vi "Custom Device CORE.vi"(8 "error in (no error)":errorcluster, 11 "CD Wizard - Internal Data":T1={"Common Information"={"CD Name"="InlineAsync", "CD Target Folder"=path "C:/Users/rsparks/Desktop/Test1", "CD Execution Mode"=enum."Inline HW Interface", "CD GUID"="", "Max Occurrences"=1}, "Extra Pages"=[{"Page Name"="Page 0", "Page GUID"="0-000000000000000-00000000000-000"}, {"Page Name"="Page11", "Page GUID"=""}, {"Page Name"="Page 2", "Page GUID"="22222222-222222222-2222222"}, {"Page Name"="Page33", "Page GUID"=""}, {"Page Name"="Page4", "Page GUID"="44444444-44444444444-4444444"}], "References"={"System Explorer Library"=refnum, "Shared Library"=refnum, "Engine Library"=refnum}, "Menu Settings"={"Insert CD in submenu"=FALSE, "Parent Menu Name"=""}}) -> (0 "error out":errorcluster)   [LabVIEW 2015]
doc: "This VI is the Core VI for the Custom Device Wizard.\n\nWritten by:\nStephan Daunke\n\nDate:\n2014/01/27\n\nCompany:\nNational Instruments Germany GmbH"
uses:
  TypDef/CD Wizard - Internal data.ctl
  TypDef/CD Wizard - Execution Mode.ctl
  TypDef/CD Wizard - Extra Page Name and GUID.ctl
  TypDef/CD Wizard - Action.ctl
  Constants/Constants TypDef/Common.ctl
  Constants/Constants TypDef/Utility folder.ctl
  Constants/Constants TypDef/CD Shared lvlib.ctl
  TypDef/Add Item - Type.ctl
  Constants/Constants TypDef/CD System Explorer lvlib.ctl
  Constants/Constants TypDef/CD Engine lvlib.ctl
  Constants/Constants TypDef/Build Spec System Explorer.ctl
  Constants/Constants TypDef/Build Spec Engine.ctl
  Constants/Common.vi
  Constants/Utility folder.vi
  Constants/CD Shared lvlib.vi
  Constants/CD System Explorer lvlib.vi
  Constants/CD Engine lvlib.vi
  <vilib>/Utility/config.llb/Write Key (String).vi
  <vilib>/Utility/config.llb/Write Key (Path).vi
  Constants/Build Spec System Explorer.vi
  Constants/Build Spec Engine.vi
  <vilib>/Utility/config.llb/NI_LVConfig.lvlib
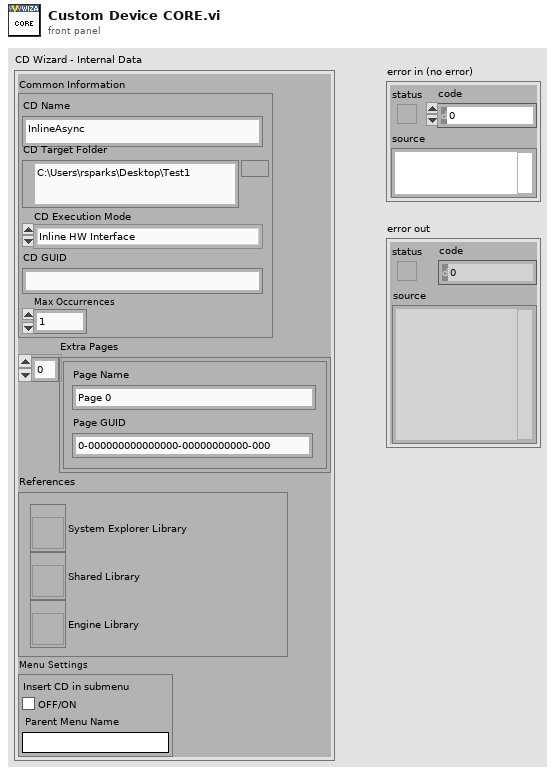
[diagram p1: front panel]
types:
  T1 = typedef "CD Wizard - Internal data.ctl" = cluster{"Common Information":cluster{"CD Name":string, "CD Target Folder":path, "CD Execution Mode":T2, "CD GUID":string, "Max Occurrences":u32}, "Extra Pages":T3[], "References":cluster{"System Explorer Library":refnum<vi>, "Shared Library":refnum<vi>, "Engine Library":refnum<vi>}, "Menu Settings":cluster{"Insert CD in submenu":bool, "Parent Menu Name":string}}
  T2 = typedef "CD Wizard - Execution Mode.ctl" = enum16{"Asynchronous", "Inline HW Interface", "Inline Model Interface", "Inline Timing and Sync", "Asynchronous Timing and Sync"}
  T3 = typedef "CD Wizard - Extra Page Name and GUID.ctl" = cluster{"Page Name":string, "Page GUID":string}
  T4 = typedef "CD Wizard - Action.ctl" = enum16{"Initialize", "Project - Create Custom Device folder", "Project - Copy Readme.rtf into the CD folder", "PC - Create GUID for each extra page", "PC-Utility - Create folder and copy -Copy .LLB to NI VeriStand dir-", "PC-Utility - Change -Copy .LLB to NI VeriStand dir-", "PC-Shared - Create folder and copy Constants.vi", "PC-Shared - Change Constants.vi content", "PC-Shared - Create library", "PC-Shared - Add folders and VIs to library", "PC-System Explorer - Create folder and copy templates", "PC-System Explorer - Create extra pages", "PC-System Explorer - Create library", "PC-System Explorer - Add folders and VIs to library", "PC-Engine - Create folder and copy the RT Template", "PC-Engine - Create library", "PC-Engine - Add virtual folders and VIs to library", "PC-XML - Create and change file", "PC-Help - Copy HTML Files", "Project - Read project file content", "Project - Edit Utility section", "Project - Edit XML section", "Project - Edit Engine Library section", "Project - Edit Shared Library section", "Project - Edit System Explorer Library section", "Project - Edit Custom Device Name", "Project - Edit System Explorer LLB Name", "Project - Edit Engine LLB OS dependent file name", "Project - Write new project file", "Shutdown"}
  T5 = typedef "Common.ctl" = enum16{"ProjectName", "TemplatesFolderName", "ProjectTemplatePathAndName", "ReadmeTemplatePathAndName", "TimingAndSyncFolderName", "CustomDeviceFolderName", "PathToTemplates"}
  T6 = typedef "Utility folder.ctl" = enum16{"Utility.FolderName", "Utility.Copy .llb to NI VeriStand dir.FileName", "Utility.Copy .llb to NI VeriStand dir.FilePathAndName", "Utility.LLB Pre Build.FilePathAndName"}
  T7 = typedef "CD Shared lvlib.ctl" = enum16{"LibraryFileName", "LibraryFolderName", "ConstantsVI.VIPathAndName", "Shared.FolderName", "Shared.Types.FolderName", "Shared.Constants.VIName", "Shared.Constants.VITemplateName", "Shared.Constants.VITemplatePathAndName", "Shared.CompiledSettings.RelativePath", "Shared.Constants.RelativePath", "Shared.CompiledSettings.Name", "Shared.CompiledSettings.Name.NoExtension", "Shared.CompiledSettings.ClusterName"}
  T8 = typedef "CD System Explorer lvlib.ctl" = enum16{"LibraryFileName", "LibraryFolderName", "System Explorer.FolderName", "System Explorer.Dynamically Called.FolderName", "System Explorer.Dynamically Called.Extra Pages.FolderName", "System Explorer.Dynamically Called.Extra Pages.TemplatePathAndName", "System Explorer.Dynamically Called.Main Page.VIName", "System Explorer.Dynamically Called.Main Page.TemplatePathAndName", "System Explorer.Dynamically Called.Initialization VI.VIName", "System Explorer.Dynamically Called.Initialization VI.TemplatePathAndName", "System Explorer.SubVI.FolderName", "System Explorer.Types.FolderName", "System Explorer.ActionVIOnCompile.VIName", "System Explorer.ExportConfigRTM.VIName"}
  T9 = typedef "CD Engine lvlib.ctl" = enum16{"LibraryFileName", "LibraryFolderName", "Engine.FolderName", "Engine.Init.FolderName", "Engine.Run.FolderName", "Engine.Shutdown.FolderName", "Types.FolderName", "Engine.RT Driver VI.TemplatePath", "Engine.RT Driver VI.FileName", "Engine.RTStateVariables.Name", "Engine.RTStateVariables.Name.NoExtension", "Engine.Async.NameExtension", "Engine.Async.TemplateName"}
  T10 = typedef "Build Spec System Explorer.ctl" = enum16{"Destinations.LLBFileName"}
  T11 = typedef "Build Spec Engine.ctl" = enum16{"Destinations.LLBWindowsFileName", "Destinations.LLBVxWorksFileName", "Destinations.LLBPharlapFileName", "Destinations.LLBLinuxARMFileName", "Destinations.LLBLinux64FileName"}
  T12 = enum16{"open", "replace", "create", "open or create", "replace or create", "replace or create with confirmation"}
  T13 = typedef "Add Item - Type.ctl" = string
  T14 = typedef "NI_LVConfig.lvlib/Config Data RefNum.ctl" = refnum<k1>
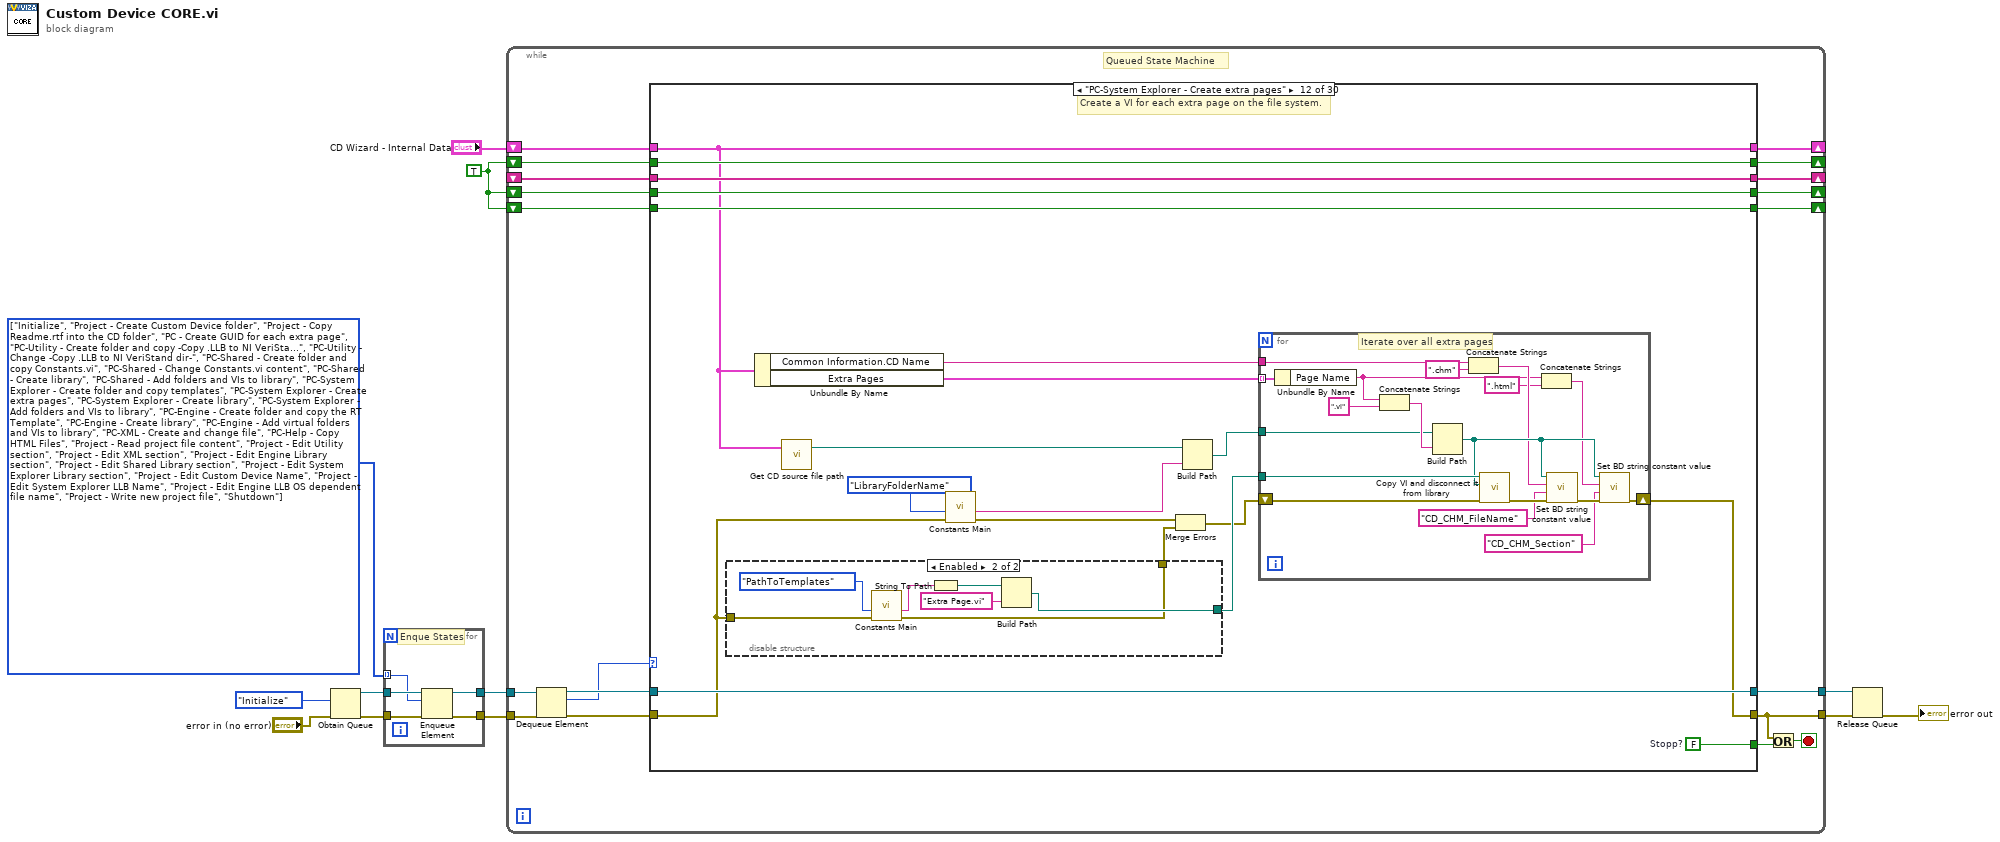
[diagram p0: block diagram]
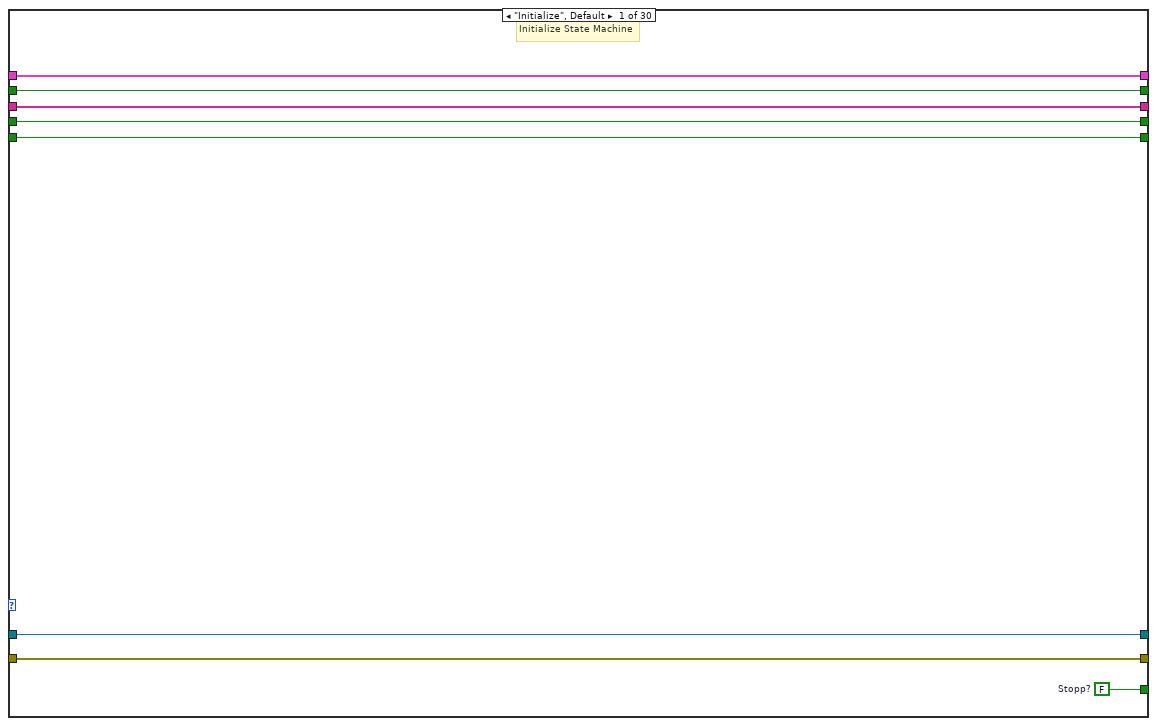
[diagram p2: hidden frame]
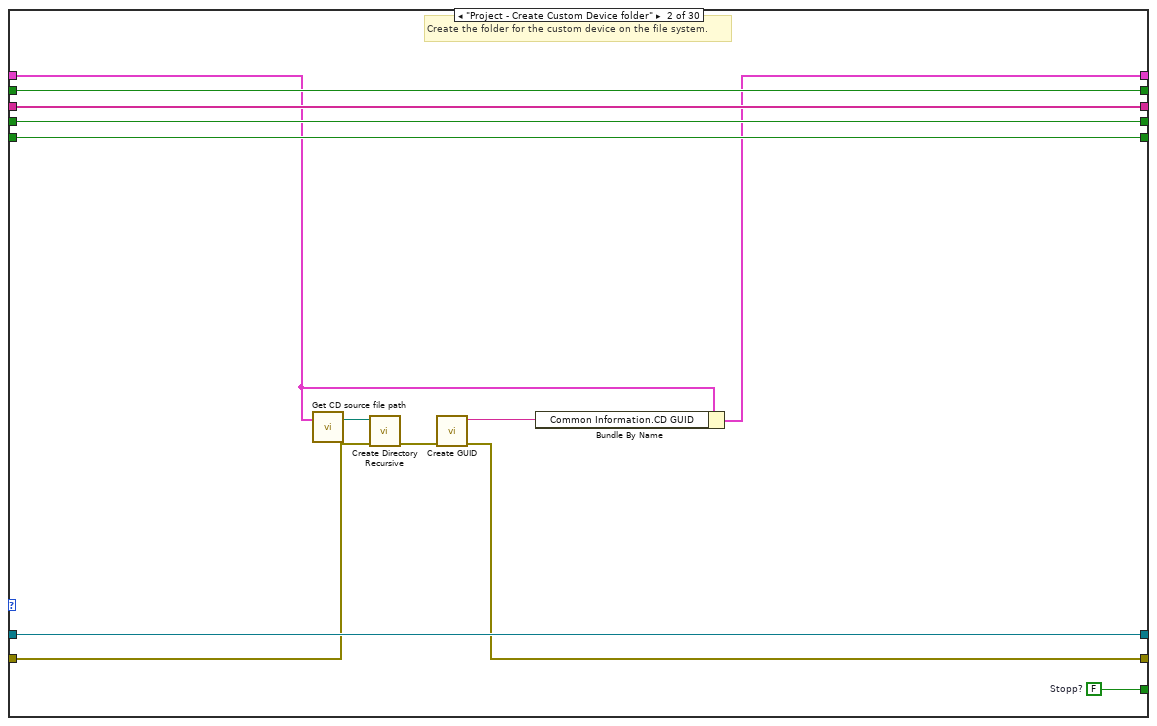
[diagram p3: hidden frame]
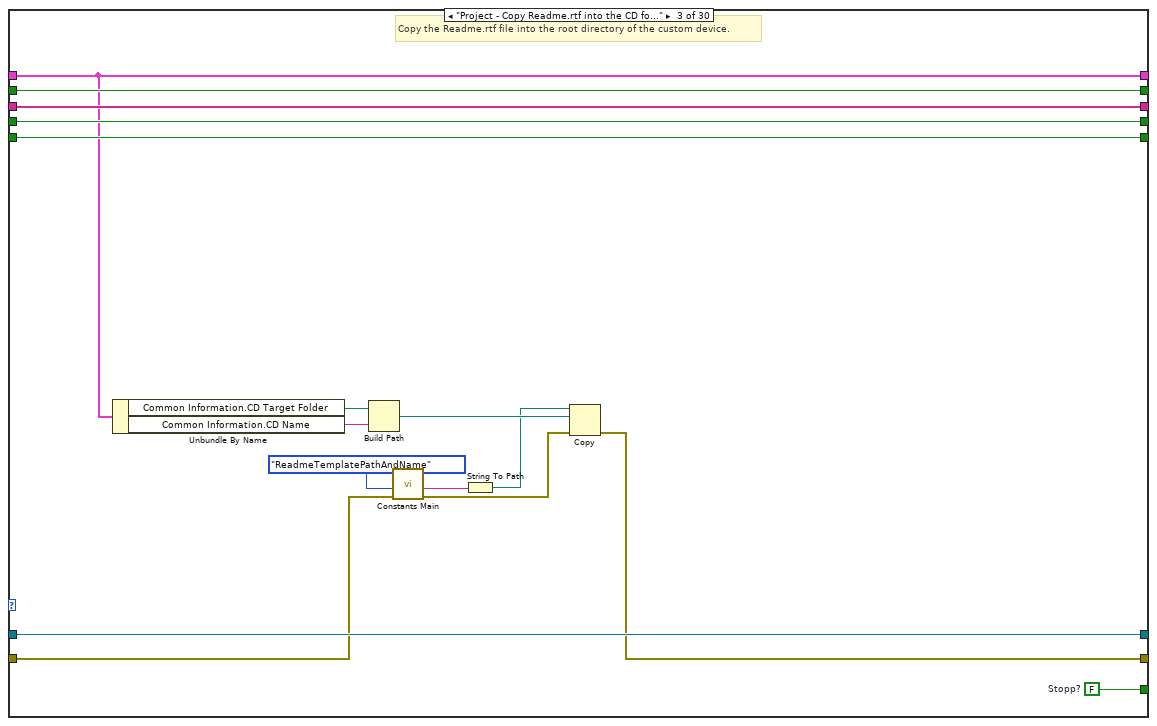
[diagram p4: hidden frame]
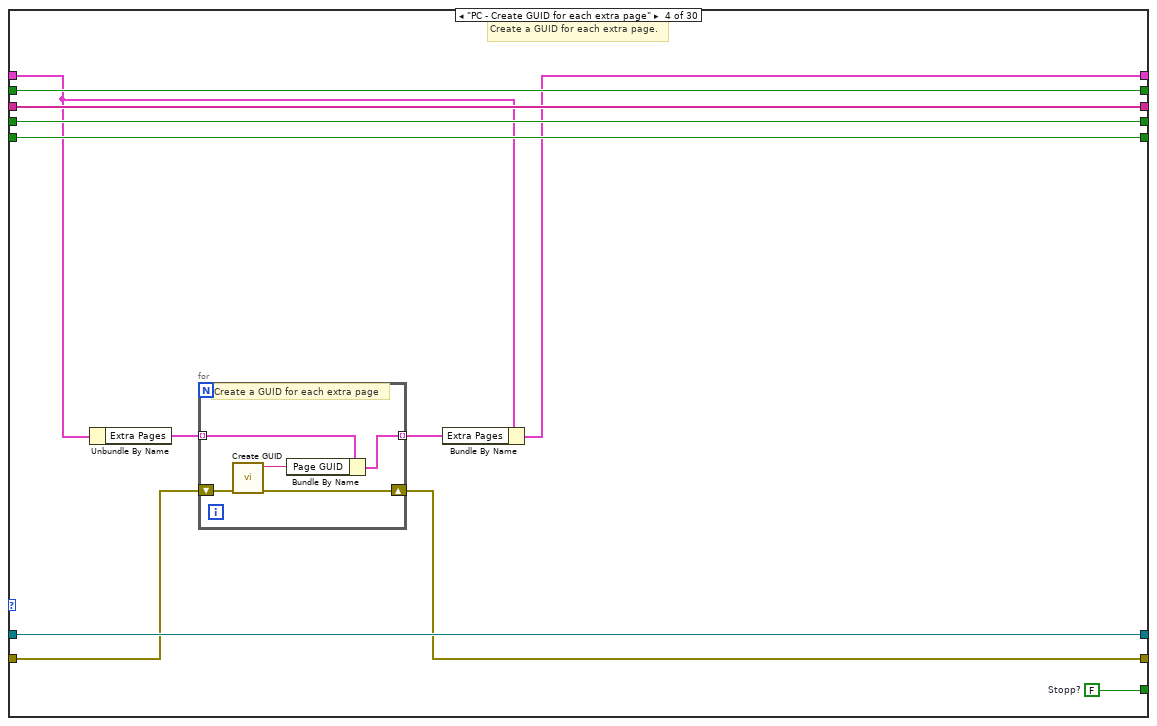
[diagram p5: hidden frame]
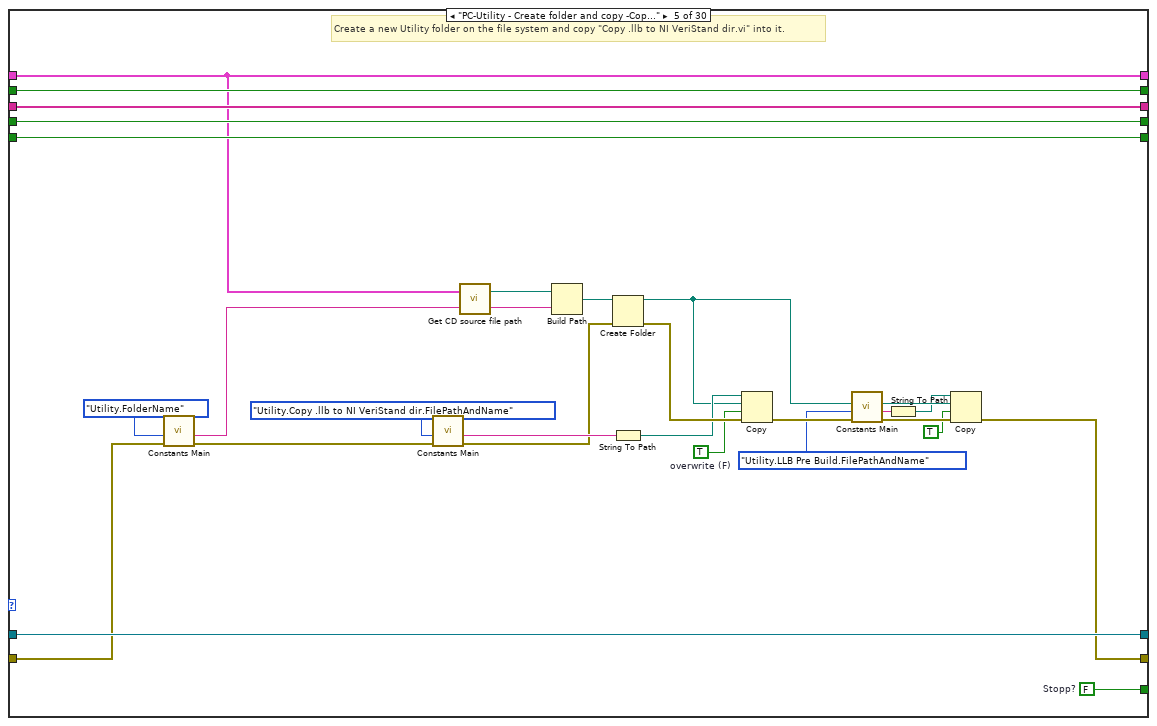
[diagram p6: hidden frame]
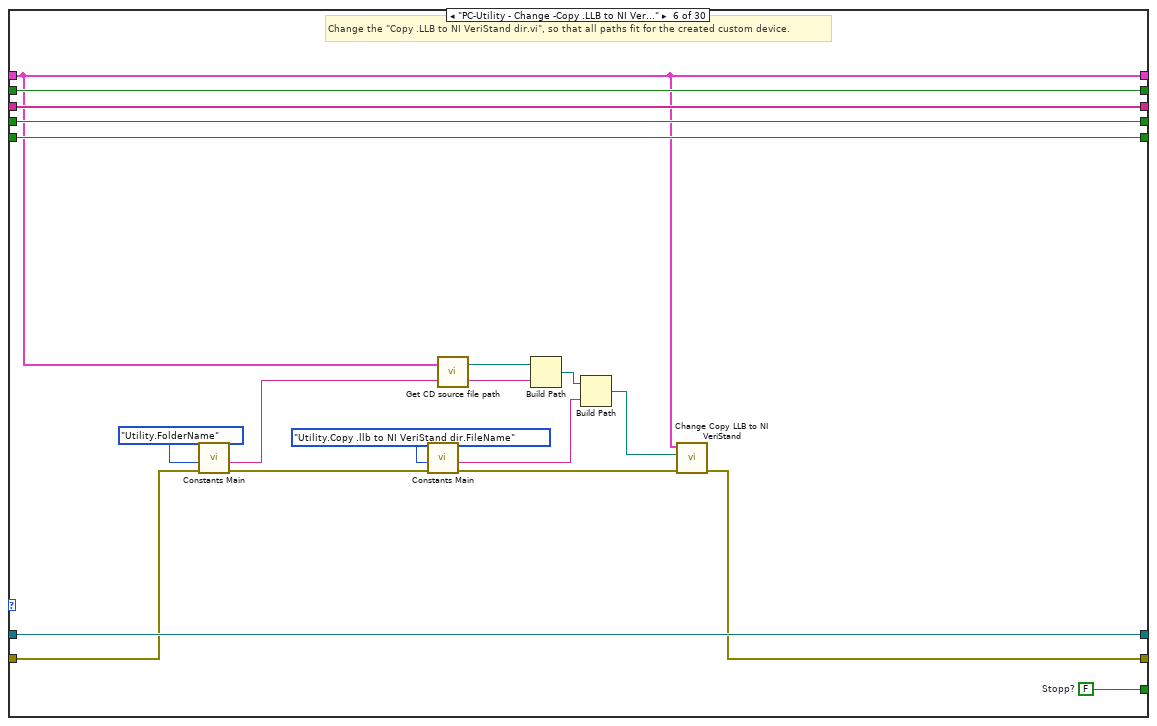
[diagram p7: hidden frame]
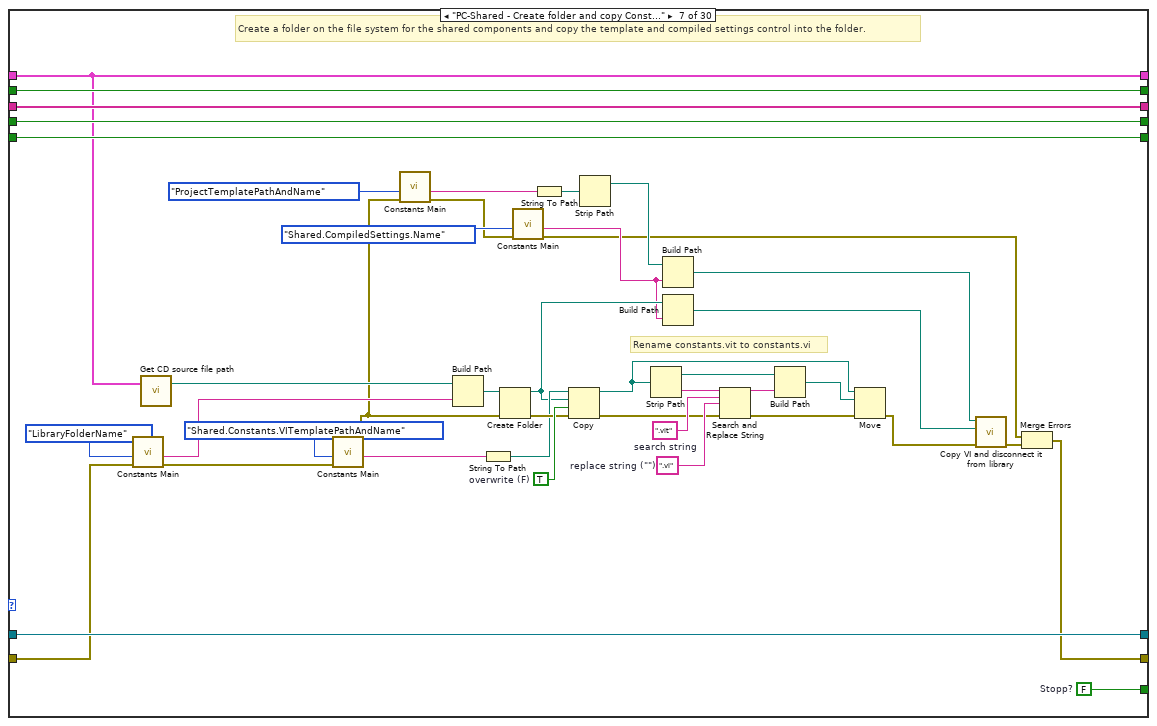
[diagram p8: hidden frame]
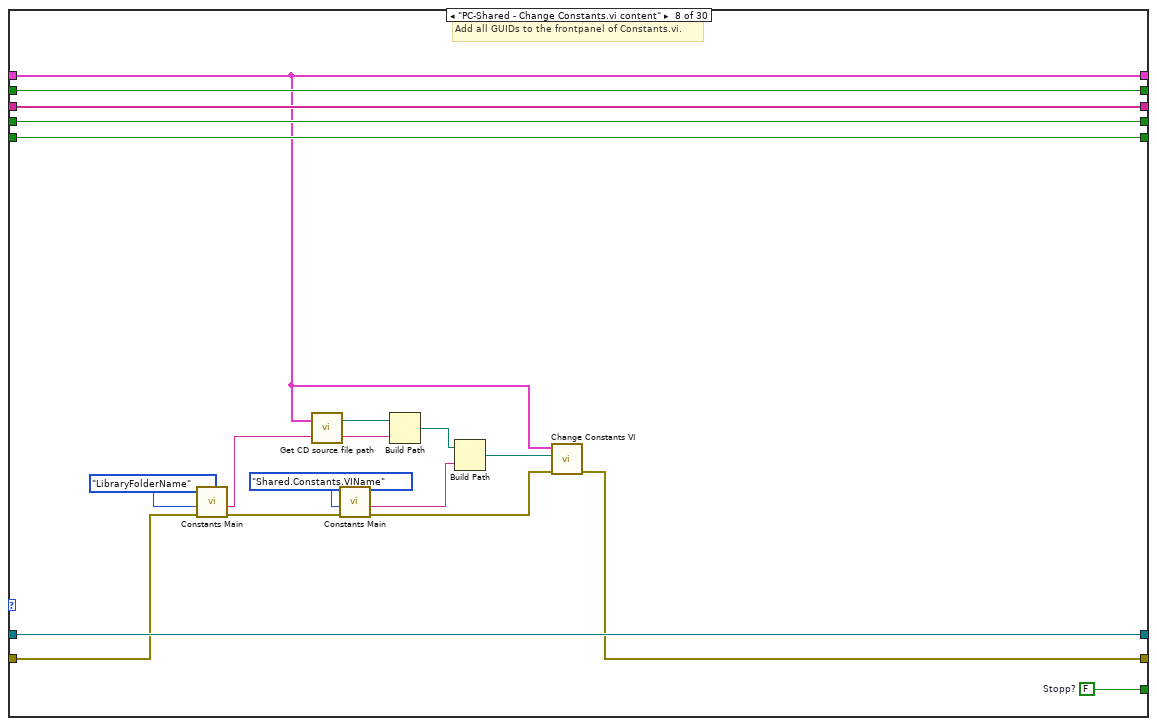
[diagram p9: hidden frame]
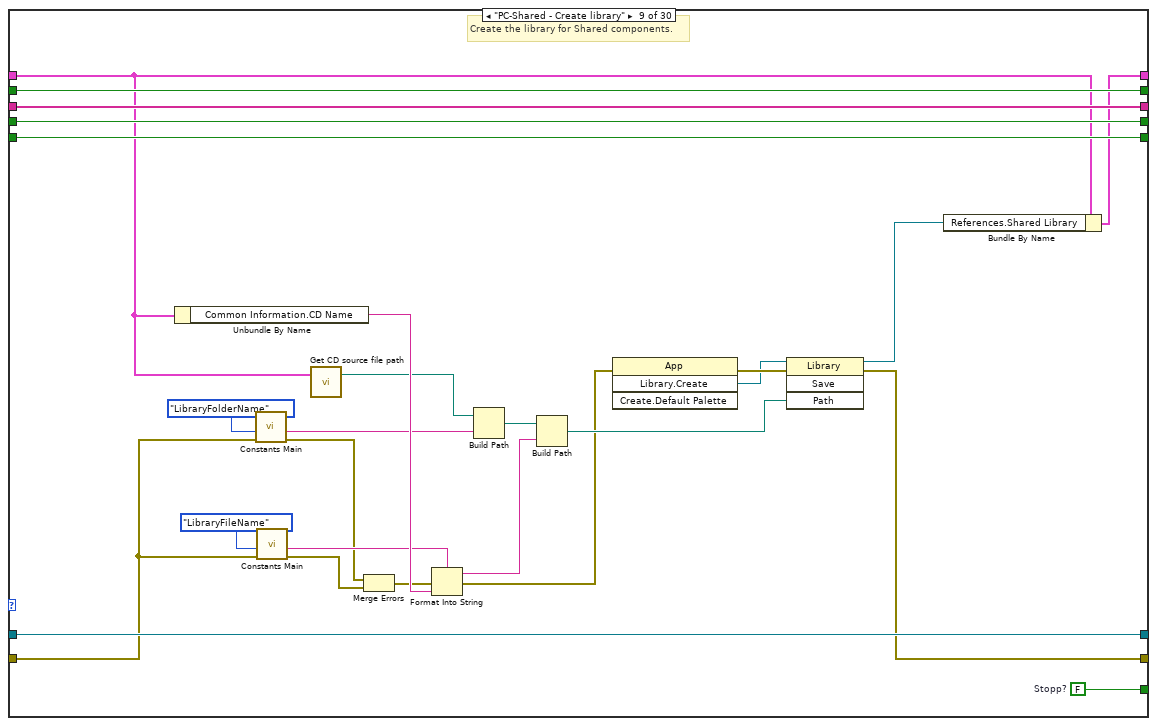
[diagram p10: hidden frame]
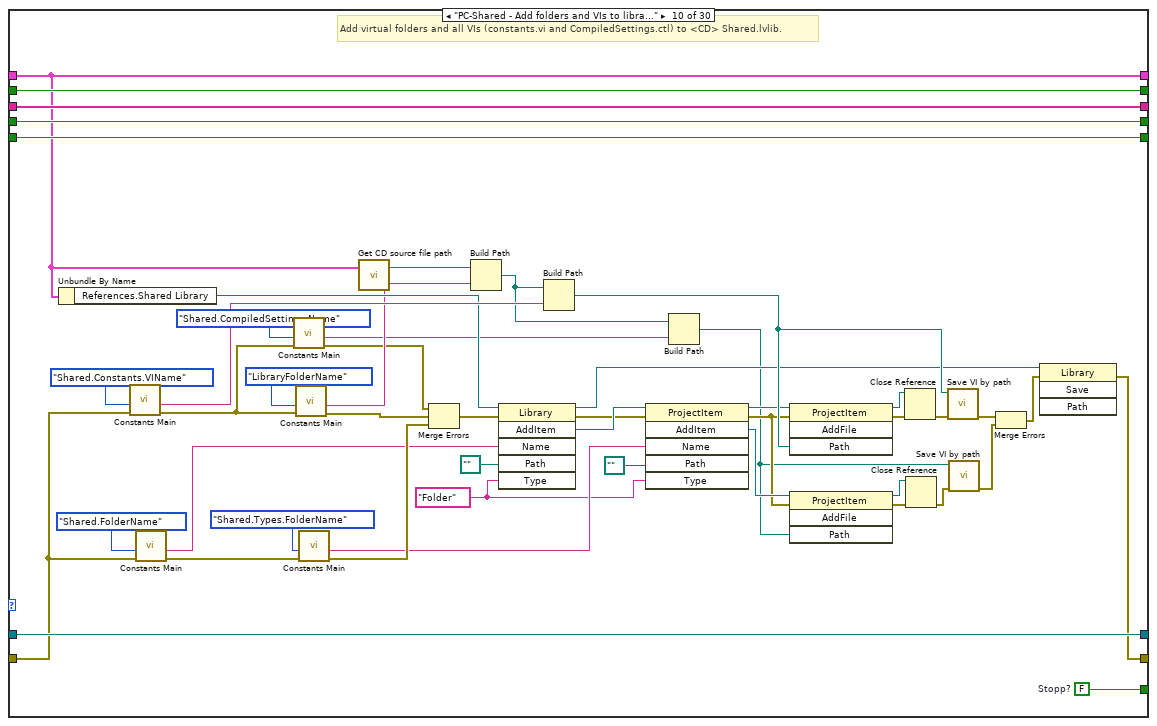
[diagram p11: hidden frame]
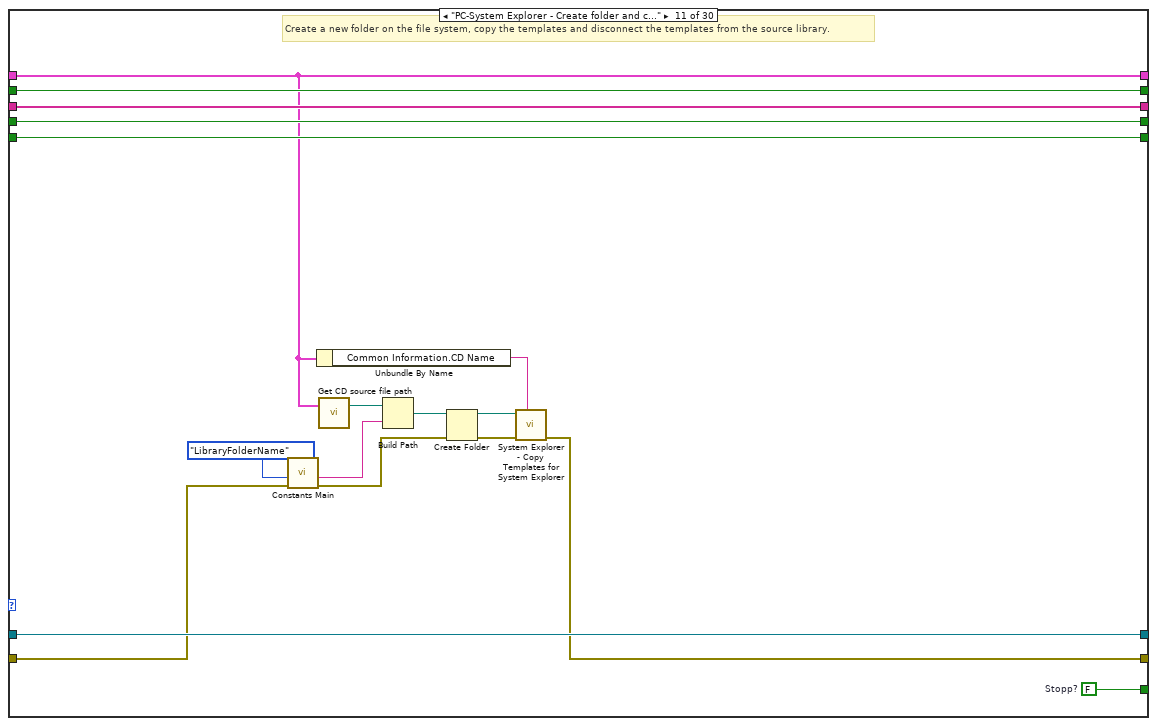
[diagram p12: hidden frame]
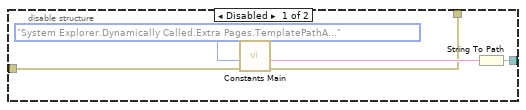
[diagram p13: hidden frame]
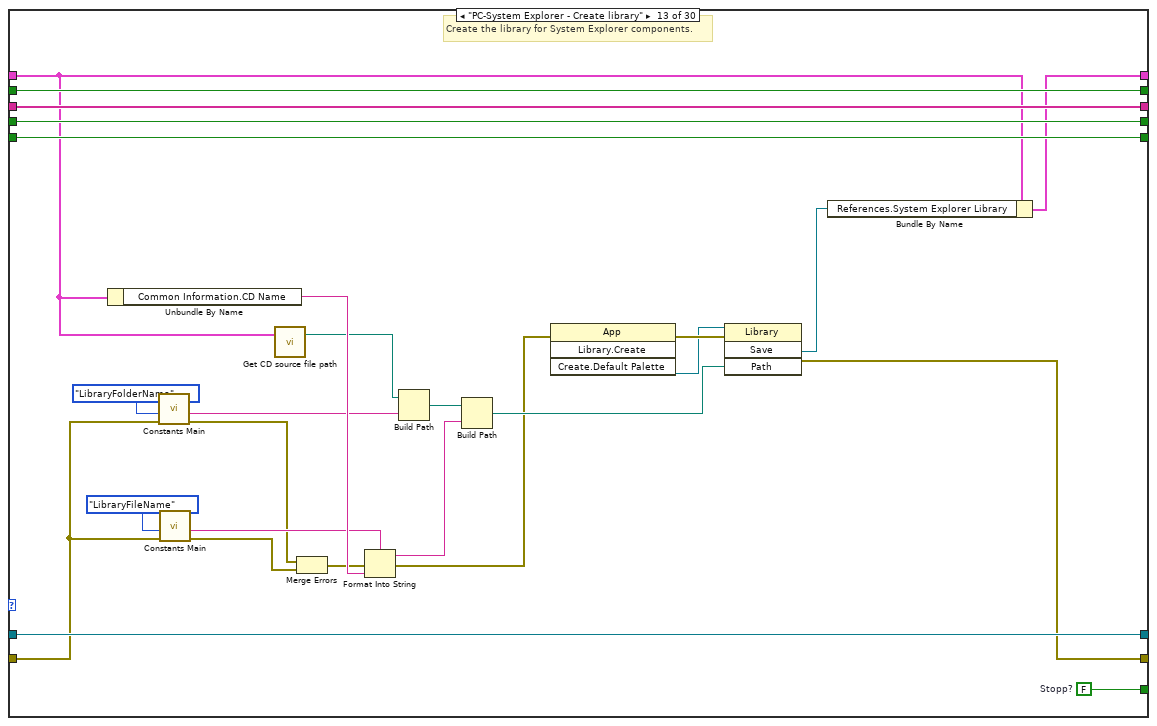
[diagram p14: hidden frame]
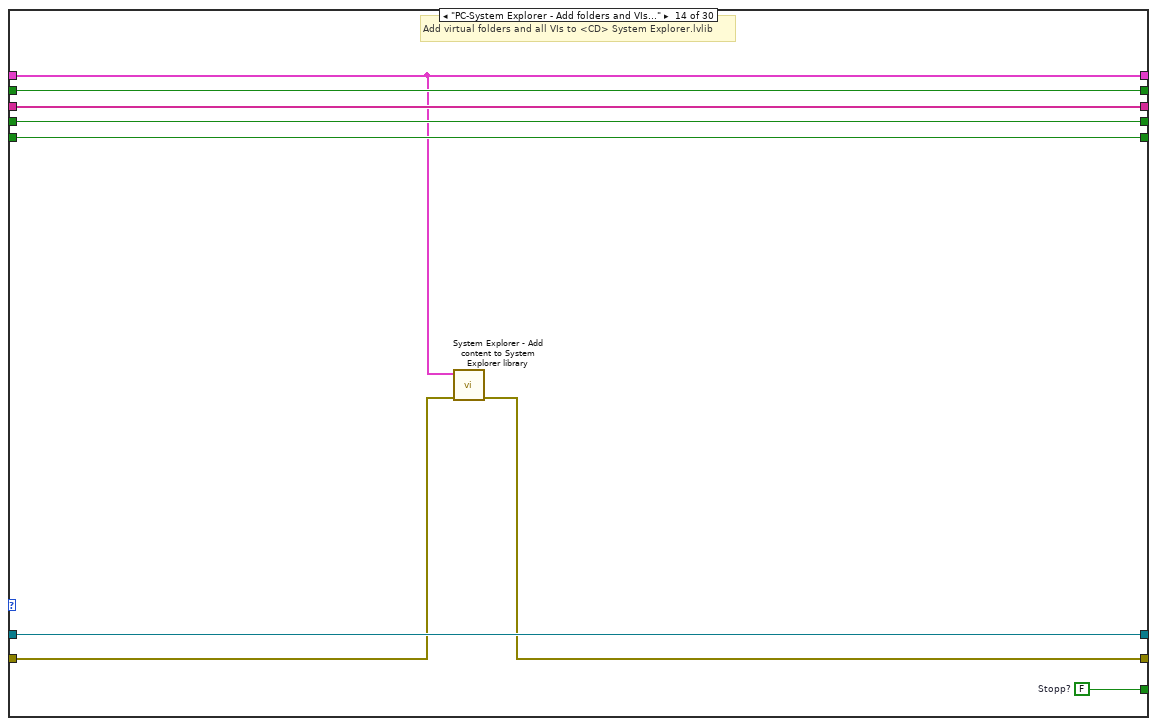
[diagram p15: hidden frame]
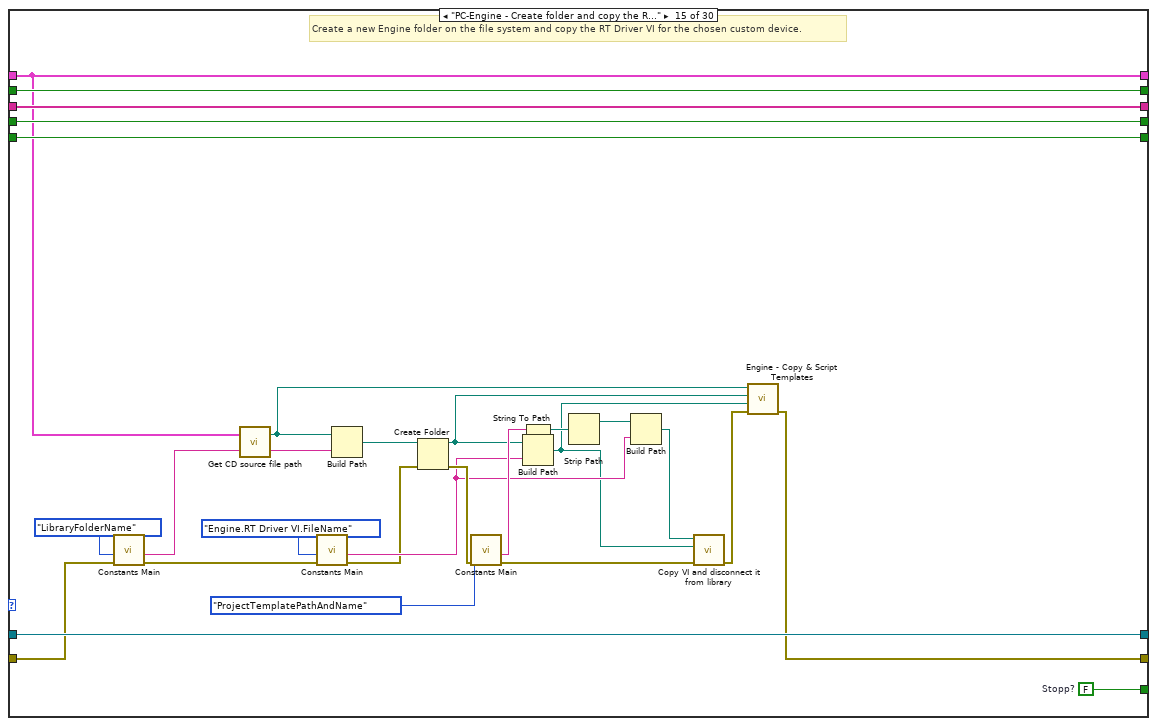
[diagram p16: hidden frame]
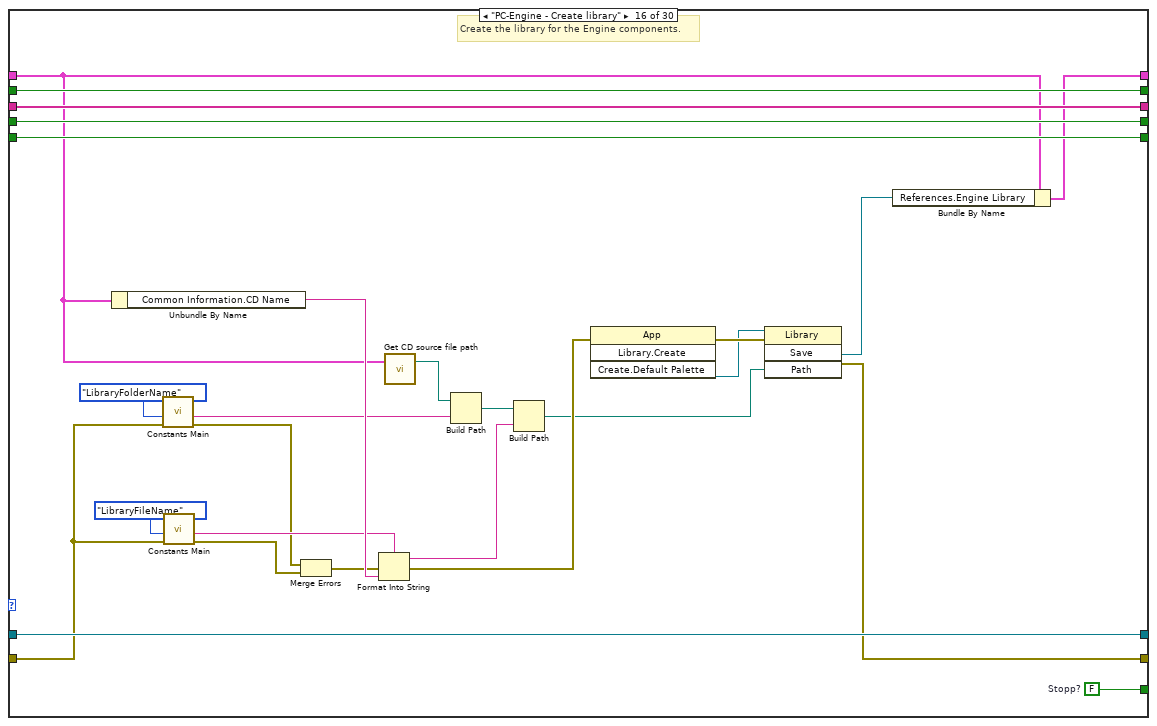
[diagram p17: hidden frame]
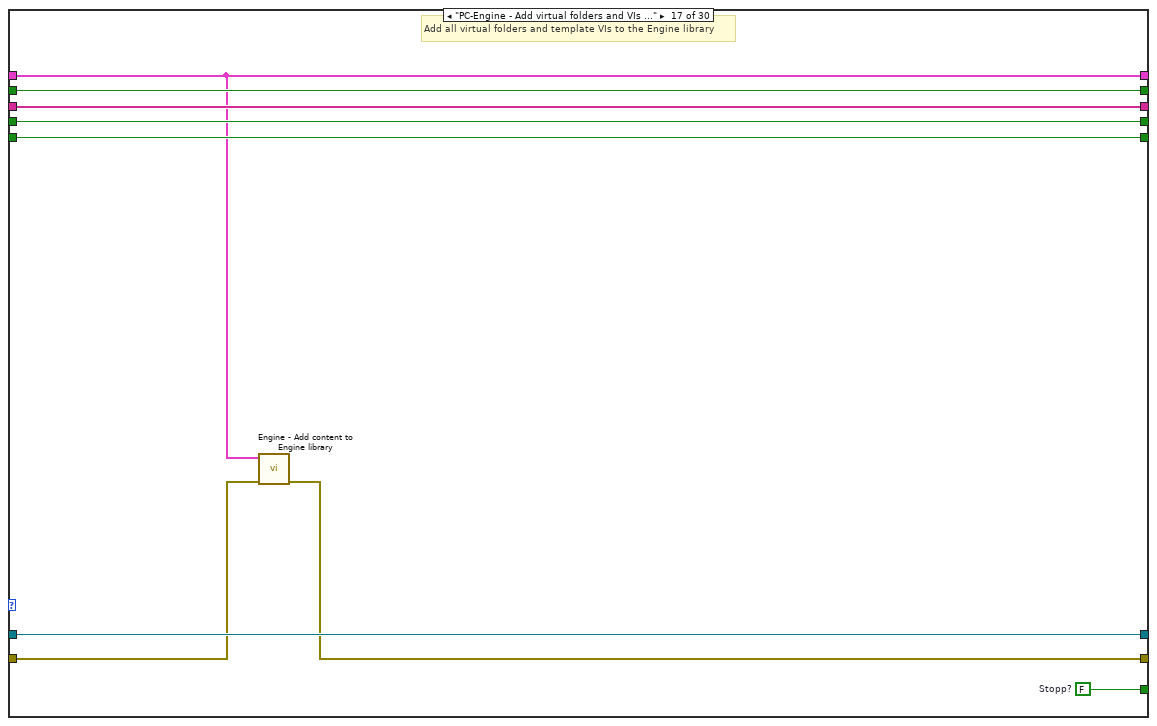
[diagram p18: hidden frame]
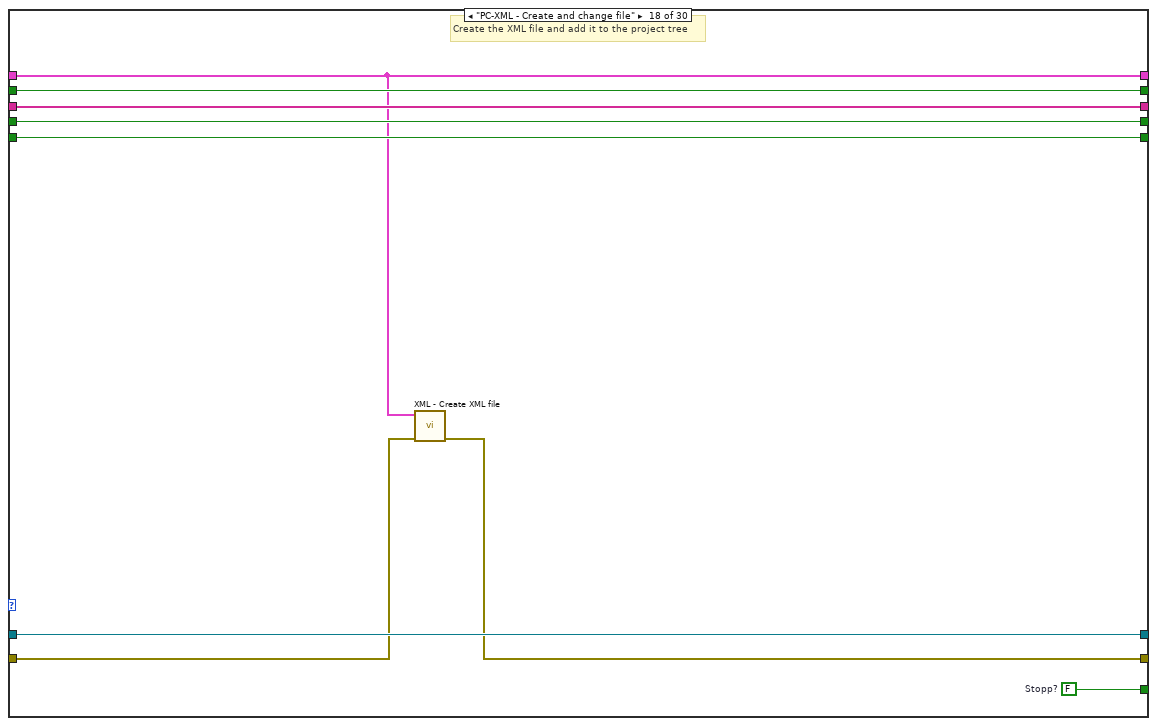
[diagram p19: hidden frame]
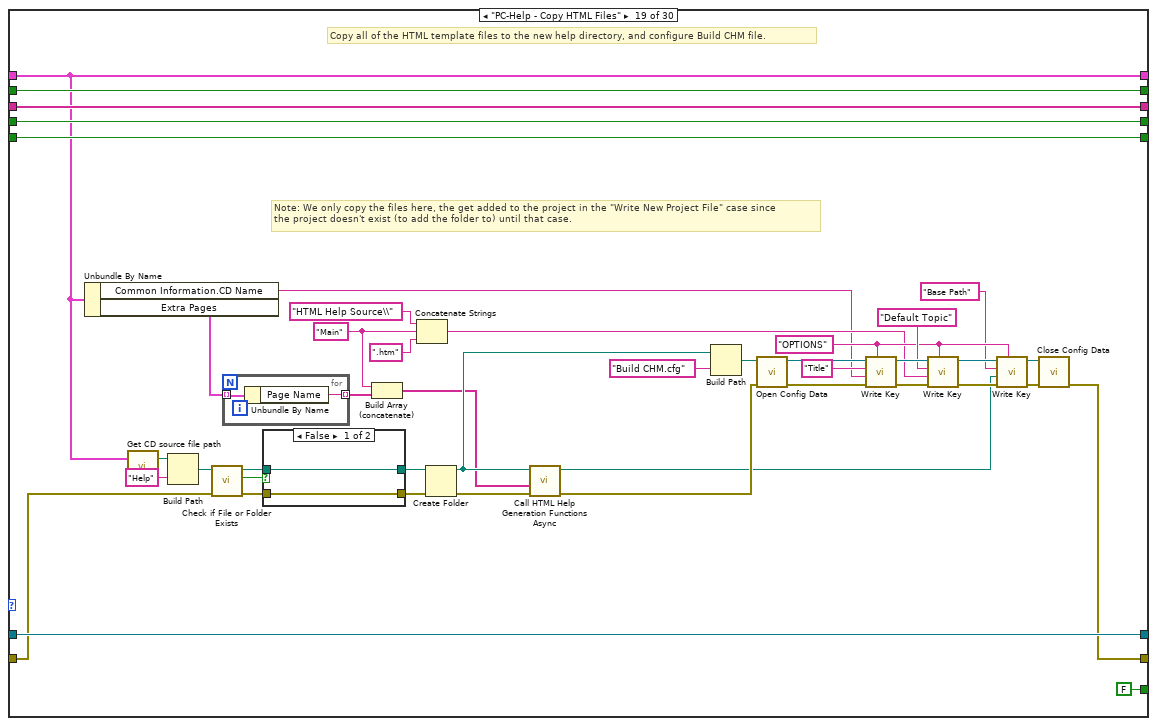
[diagram p20: hidden frame]
diagram:
  w3 = TRUE
  w6 = T4[] [enum."Initialize", enum."Project - Create Custom Device folder", enum."Project - Copy Readme.rtf into the CD folder", enum."PC - Create GUID for each extra page", enum."PC-Utility - Create folder and copy -Copy .LLB to NI VeriStand dir-", enum."PC-Utility - Change -Copy .LLB to NI VeriStand dir-", enum."PC-Shared - Create folder and copy Constants.vi", enum."PC-Shared - Change Constants.vi content", enum."PC-Shared - Create library", enum."PC-Shared - Add folders and VIs to library", enum."PC-System Explorer - Create folder and copy templates", enum."PC-System Explorer - Create extra pages", enum."PC-System Explorer - Create library", enum."PC-System Explorer - Add folders and VIs to library", enum."PC-Engine - Create folder and copy the RT Template", enum."PC-Engine - Create library", enum."PC-Engine - Add virtual folders and VIs to library", enum."PC-XML - Create and change file", enum."PC-Help - Copy HTML Files", enum."Project - Read project file content", enum."Project - Edit Utility section", enum."Project - Edit XML section", enum."Project - Edit Engine Library section", enum."Project - Edit Shared Library section", enum."Project - Edit System Explorer Library section", enum."Project - Edit Custom Device Name", enum."Project - Edit System Explorer LLB Name", enum."Project - Edit Engine LLB OS dependent file name", enum."Project - Write new project file", enum."Shutdown"] items=["Initialize", "Project - Create Custom Device folder", "Project - Copy Readme.rtf into the CD folder", "PC - Create GUID for each extra page", "PC-Utility - Create folder and copy -Copy .LLB to NI VeriStand dir-", "PC-Utility - Change -Copy .LLB to NI VeriStand dir-", "PC-Shared - Create folder and copy Constants.vi", "PC-Shared - Change Constants.vi content", "PC-Shared - Create library", "PC-Shared - Add folders and VIs to library", "PC-System Explorer - Create folder and copy templates", "PC-System Explorer - Create extra pages", "PC-System Explorer - Create library", "PC-System Explorer - Add folders and VIs to library", "PC-Engine - Create folder and copy the RT Template", "PC-Engine - Create library", "PC-Engine - Add virtual folders and VIs to library", "PC-XML - Create and change file", "PC-Help - Copy HTML Files", "Project - Read project file content", "Project - Edit Utility section", "Project - Edit XML section", "Project - Edit Engine Library section", "Project - Edit Shared Library section", "Project - Edit System Explorer Library section", "Project - Edit Custom Device Name", "Project - Edit System Explorer LLB Name", "Project - Edit Engine LLB OS dependent file name", "Project - Write new project file", "Shutdown"]
  n1 = Obtain Queue(element data type=CD_Wizard_-_Action."Initialize", error in (no error)="error in (no error)") -> (queue out=w10:refnum<queue>, error out=w9:errorcluster)  [unwired: 3 in, 1 out]
  n2 = for {
    tunnel: w10 -> [w17]
    tunnel: w9 -> [w16]
    tunnel: [w15] -> w8
    tunnel: [w14] -> w7
    tunnel: w6 -> [w13] mode=indexing
    # "Enque States"
    n3 = Enqueue Element(queue=w17, element=w13, error in (no error)=w16) -> (queue out=w15:refnum<queue>, error out=w14:errorcluster)  [unwired: 1 in, 1 out]
  }
  n4 = while {
    tunnel: w8 -> [w36]
    tunnel: w7 -> [w35]
    tunnel: [w21] -> w4
    tunnel: [w32] -> w11
    shift-right: [w27] -> _
    shift-left: "CD Wizard - Internal Data" -> [w31]
    shift-right: [w26] -> _
    shift-left: w3 -> [w30]
    shift-right: [w25] -> _
    shift-left: _ -> [w29]
    shift-right: [w24] -> _
    shift-left: w3 -> [w28]
    shift-right: [w23] -> _
    shift-left: w3 -> [w20]
    stop <- w22 stop-if-true
    # "Queued State Machine"
    n5 = Dequeue Element(queue=w36, error in (no error)=w35) -> (queue out=w34:refnum<queue>, element=w19:T4, error out=w33:errorcluster)  [unwired: 1 in, 1 out]
    n6 = case shown="\"PC-System Explorer - Create extra pages\"" w19 {
      tunnel: w34 -> [w44 w57 w73 w85 w117 w135 w177 w195 w221 w269 w286 w305 w361 w370 w397 w423 w432 w441 w484 w511 w533 w563 w581 w604 w643 w670 w694 w740 w791 w799]
      tunnel: w33 -> [w39 w47 w62 w79 w102 w123 w171 w181 w198 w241 w278 w289 w345 w365 w383 w405 w427 w436 w457 w497 w516 w555 w576 w587 w622 w666 w686 w712 w782 w798]
      tunnel: [w44 w57 w73 w85 w117 w135 w177 w195 w221 w269 w286 w305 w361 w370 w397 w423 w432 w441 w484 w511 w533 w563 w581 w604 w643 w670 w694 w740 w791 w799] -> w32
      tunnel: [w39 w50 w64 w78 w91 w122 w137 w190 w197 w240 w274 w299 w337 w364 w374 w401 w426 w435 w456 w502 w526 w559 w575 w599 w626 w665 w690 w721 w772 w798] -> w21
      tunnel: w31 -> [w38 w49 w66 w76 w100 w120 w165 w179 w201 w242 w271 w298 w343 w363 w387 w407 w425 w434 w452 w508 w529 w556 w574 w583 w623 w661 w684 w733 w783 w797]
      tunnel: w30 -> [w43 w56 w72 w84 w116 w134 w176 w194 w220 w268 w285 w304 w360 w369 w396 w422 w431 w440 w483 w495 w532 w562 w580 w603 w642 w669 w693 w739 w788 w796]
      tunnel: w29 -> [w42 w55 w71 w83 w115 w133 w175 w193 w219 w267 w284 w303 w359 w368 w395 w421 w430 w439 w482 _ w528 w558 w573 w588 w624 w663 w681 w722 w775 w795]
      tunnel: w28 -> [w40 w54 w70 w82 w114 w132 w174 w192 w218 w266 w283 w302 w358 w367 w394 w420 w429 w438 w481 w510 w531 w561 w579 w602 w641 w668 w692 w738 w790 w794]
      tunnel: w20 -> [w41 w53 w69 w81 w113 w131 w173 w191 w217 w265 w282 w301 w357 w366 w393 w419 w428 w437 w480 w509 w530 w560 w578 w601 w640 w667 w691 w737 w789 w793]
      tunnel: [w38 w52 w66 w75 w100 w120 w165 w179 w200 w242 w271 w298 w346 w363 w387 w406 w425 w434 w452 w508 w529 w556 w574 w583 w623 w661 w684 w733 w783 w797] -> w27
      tunnel: [w43 w56 w72 w84 w116 w134 w176 w194 w220 w268 w285 w304 w360 w369 w396 w422 w431 w440 w483 w495 w532 w562 w580 w603 w642 w669 w693 w739 w788 w796] -> w26
      tunnel: [w42 w55 w71 w83 w115 w133 w175 w193 w219 w267 w284 w303 w359 w368 w395 w421 w430 w439 w482 w501 w527 w557 w577 w600 w625 w664 w680 w703 w775 w795] -> w25
      tunnel: [w40 w54 w70 w82 w114 w132 w174 w192 w218 w266 w283 w302 w358 w367 w394 w420 w429 w438 w481 w510 w531 w561 w579 w602 w641 w668 w692 w738 w790 w794] -> w24
      tunnel: [w41 w53 w69 w81 w113 w131 w173 w191 w217 w265 w282 w301 w357 w366 w393 w419 w428 w437 w480 w509 w530 w560 w578 w601 w640 w667 w691 w737 w789 w793] -> w23
      tunnel: [w37 w45 w58 w74 w99 w118 w163 w178 w196 w235 w272 w288 w336 w362 w382 w398 w424 w433 FALSE ("Stopp?") w494 w518 w550 w572 w582 w621 w660 w679 w720 w770 w792] -> w18
      frame "Initialize", Default {
        w37 = FALSE  # Stopp?
        # "Initialize State Machine"
      }
      frame "Project - Create Custom Device folder" {
        w45 = FALSE  # Stopp?
        # "Create the folder for the custom device on the file system."
        n7 = call "Get CD source file path.vi"("CD Wizard - Internal Data"=w49) -> ("CD Source file path"=w48:path)  [unwired: 2 in]
        n8 = call <vilib>:"Create Directory Recursive.vi"("error in (no error)"=w47, "directory"=w48) -> ("error out"=w46:errorcluster)  [unwired: 3 in, 2 out]
        n9 = call "Create GUID.vi"("error in (no error)"=w46) -> ("error out"=w50:errorcluster, "Generated GUID"=w51:string)  [unwired: 9 in]
        n10 = Bundle By Name(cluster=w49, "Common Information.CD GUID"=w51) -> (w52:T1)
      }
      frame "Project - Copy Readme.rtf into the CD folder" {
        w58 = FALSE  # Stopp?
        # "Copy the Readme.rtf file into the root directory of the custom device."
        n11 = Unbundle By Name(w66) -> ("Common Information.CD Target Folder"=w68:path, "Common Information.CD Name"=w67:string)
        n12 = Build Path(base path=w68, name or relative path=w67) -> (appended path=w65:path)
        n13 = call-poly "Constants Main.vi"("error in (no error)"=w62, "Action"=Common."ReadmeTemplatePathAndName") -> ("error out"=w61:errorcluster, "Output"=w60:string)  [unwired: 8 in]
        n14 = String To Path(string=w60) -> (path=w59:path)
        n15 = Copy(8:w61, 10:w65, 11:w59) -> (0:w64:errorcluster)  [unwired: 1 in, 3 out]
      }
      frame "PC - Create GUID for each extra page" {
        w74 = FALSE  # Stopp?
        # "Create a GUID for each extra page."
        n16 = Unbundle By Name(w76) -> ("Extra Pages"=w80:T3[])
        n17 = for {
          tunnel: w80 -> [w90] mode=indexing
          shift-right: [w87] -> w78
          shift-left: w79 -> [w88]
          tunnel: [w86] -> w77 mode=indexing
          # "Create a GUID for each extra page"
          n18 = call "Create GUID.vi"("error in (no error)"=w88) -> ("error out"=w87:errorcluster, "Generated GUID"=w89:string)  [unwired: 9 in]
          n19 = Bundle By Name(cluster=w90, "Page GUID"=w89) -> (w86:T3)
        }
        n20 = Bundle By Name(cluster=w76, "Extra Pages"=w77) -> (w75:T1)
      }
      frame "PC-Utility - Create folder and copy -Copy .LLB to NI VeriStand dir-" {
        w99 = FALSE  # Stopp?
        w110 = TRUE  # overwrite (F)
        # "Create a new Utility folder on the file system and copy \"Copy .llb to NI VeriStand dir.vi\" into it."
        n21 = call-poly "Constants Main.vi"("error in (no error)"=w102, "Action"=Utility_folder."Utility.FolderName") -> ("error out"=w103:errorcluster, "Output"=w104:string)  [unwired: 8 in]
        n22 = call-poly "Constants Main.vi"("error in (no error)"=w103, "Action"=Utility_folder."Utility.Copy .llb to NI VeriStand dir.FilePathAndName") -> ("error out"=w106:errorcluster, "Output"=w108:string)  [unwired: 8 in]
        n23 = call "Get CD source file path.vi"("CD Wizard - Internal Data"=w100) -> ("CD Source file path"=w101:path)  [unwired: 2 in]
        n24 = Build Path(base path=w101, name or relative path=w104) -> (appended path=w112:path)
        n25 = Create Folder(path (use dialog)=w112, error in=w106) -> (created path=w98:path, error out=w111:errorcluster)  [unwired: 1 in, 1 out]
        n26 = String To Path(string=w108) -> (path=w107:path)
        n27 = Copy(8:w111, 9:w110, 10:w98, 11:w107) -> (0:w97:errorcluster)  [unwired: 3 out]
        n28 = call-poly "Constants Main.vi"("error in (no error)"=w97, "Action"=Utility_folder."Utility.LLB Pre Build.FilePathAndName") -> ("error out"=w93:errorcluster, "Output"=w95:string)  [unwired: 8 in]
        n29 = String To Path(string=w95) -> (path=w94:path)
        n30 = Copy(8:w93, 9:TRUE ("overwrite (F)"), 10:w98, 11:w94) -> (0:w91:errorcluster)  [unwired: 3 out]
      }
      frame "PC-Utility - Change -Copy .LLB to NI VeriStand dir-" {
        w118 = FALSE  # Stopp?
        # "Change the \"Copy .LLB to NI VeriStand dir.vi\", so that all paths fit for the created custom device."
        n31 = call-poly "Constants Main.vi"("error in (no error)"=w123, "Action"=Utility_folder."Utility.FolderName") -> ("error out"=w127:errorcluster, "Output"=w128:string)  [unwired: 8 in]
        n32 = call-poly "Constants Main.vi"("error in (no error)"=w127, "Action"=Utility_folder."Utility.Copy .llb to NI VeriStand dir.FileName") -> ("error out"=w124:errorcluster, "Output"=w125:string)  [unwired: 8 in]
        n33 = call "Get CD source file path.vi"("CD Wizard - Internal Data"=w120) -> ("CD Source file path"=w119:path)  [unwired: 2 in]
        n34 = Build Path(base path=w119, name or relative path=w128) -> (appended path=w126:path)
        n35 = Build Path(base path=w126, name or relative path=w125) -> (appended path=w121:path)
        n36 = call "Change Copy LLB to NI VeriStand.vi"("error in (no error)"=w124, "Copy .LLB to ... path"=w121, "CD Wizard - Internal Data"=w120) -> ("error out"=w122:errorcluster)  [unwired: 8 in]
      }
      frame "PC-Shared - Create folder and copy Constants.vi" {
        w157 = ".vi"  # replace string ("")
        w158 = ".vit"  # search string
        w163 = FALSE  # Stopp?
        w162 = TRUE  # overwrite (F)
        # "Rename constants.vit to constants.vi"
        # "Create a folder on the file system for the shared components and copy the template and compiled settings control into the folder."
        n37 = call-poly "Constants Main.vi"("error in (no error)"=w171, "Action"=CD_Shared_lvlib."LibraryFolderName") -> ("error out"=w167:errorcluster, "Output"=w169:string)  [unwired: 8 in]
        n38 = call "Get CD source file path.vi"("CD Wizard - Internal Data"=w165) -> ("CD Source file path"=w164:path)  [unwired: 2 in]
        n39 = call-poly "Constants Main.vi"("error in (no error)"=w167, "Action"=CD_Shared_lvlib."Shared.Constants.VITemplatePathAndName") -> ("error out"=w140:errorcluster, "Output"=w166:string)  [unwired: 8 in]
        n40 = call-poly "Constants Main.vi"("error in (no error)"=w140, "Action"=Common."ProjectTemplatePathAndName") -> ("error out"=w138:errorcluster, "Output"=w149:string)  [unwired: 8 in]
        n41 = Build Path(base path=w164, name or relative path=w169) -> (appended path=w172:path)
        n42 = String To Path(string=w166) -> (path=w155:path)
        n43 = Create Folder(path (use dialog)=w172, error in=w140) -> (created path=w146:path, error out=w156:errorcluster)  [unwired: 1 in, 1 out]
        n44 = call-poly "Constants Main.vi"("error in (no error)"=w138, "Action"=CD_Shared_lvlib."Shared.CompiledSettings.Name") -> ("error out"=w136:errorcluster, "Output"=w139:string)  [unwired: 8 in]
        n45 = String To Path(string=w149) -> (path=w148:path)
        n46 = Copy(8:w156, 9:w162, 10:w146, 11:w155) -> (0:w154:errorcluster, 3:w151:path)  [unwired: 2 out]
        n47 = Strip Path(path=w148) -> (stripped path=w147:path)  [unwired: 1 out]
        n48 = Strip Path(path=w151) -> (stripped path=w161:path, name=w160:string)
        n49 = Build Path(base path=w147, name or relative path=w139) -> (appended path=w145:path)
        n50 = Build Path(base path=w146, name or relative path=w139) -> (appended path=w144:path)
        n51 = Search and Replace String(input string=w160, search string=w158, replace string=w157, error in=w154) -> (result string=w159:string, error out=w153:errorcluster)  [unwired: 4 in, 2 out]
        n52 = Build Path(base path=w161, name or relative path=w159) -> (appended path=w152:path)
        n53 = Move(source path=w151, error in=w153, 10:w152) -> (error out=w143:errorcluster)  [unwired: 2 in, 2 out]
        n54 = call "Copy VI and disconnect it from library.vi"("error in (no error)"=w143, "VI Target Path"=w144, "VI Source Path"=w145) -> ("error out"=w142:errorcluster)  [unwired: 8 in]
        n55 = Merge Errors(w136, w142) -> (w137:errorcluster)
      }
      frame "PC-Shared - Change Constants.vi content" {
        w178 = FALSE  # Stopp?
        # "Add all GUIDs to the frontpanel of Constants.vi."
        n56 = call-poly "Constants Main.vi"("error in (no error)"=w181, "Action"=CD_Shared_lvlib."LibraryFolderName") -> ("error out"=w184:errorcluster, "Output"=w183:string)  [unwired: 8 in]
        n57 = call "Get CD source file path.vi"("CD Wizard - Internal Data"=w179) -> ("CD Source file path"=w180:path)  [unwired: 2 in]
        n58 = call-poly "Constants Main.vi"("error in (no error)"=w184, "Action"=CD_Shared_lvlib."Shared.Constants.VIName") -> ("error out"=w182:errorcluster, "Output"=w186:string)  [unwired: 8 in]
        n59 = Build Path(base path=w180, name or relative path=w183) -> (appended path=w189:path)
        n60 = Build Path(base path=w189, name or relative path=w186) -> (appended path=w188:path)
        n61 = call "Change Constants VI.vi"("error in (no error)"=w182, "Constants.vi path"=w188, "CD Wizard - Internal Data"=w179) -> ("error out"=w190:errorcluster)  [unwired: 8 in]
      }
      frame "PC-Shared - Create library" {
        w196 = FALSE  # Stopp?
        # "Create the library for Shared components."
        n62 = Unbundle By Name(w201) -> ("Common Information.CD Name"=w216:string)
        n63 = call-poly "Constants Main.vi"("error in (no error)"=w198, "Action"=CD_Shared_lvlib."LibraryFolderName") -> ("error out"=w209:errorcluster, "Output"=w210:string)  [unwired: 8 in]
        n64 = call-poly "Constants Main.vi"("error in (no error)"=w198, "Action"=CD_Shared_lvlib."LibraryFileName") -> ("error out"=w207:errorcluster, "Output"=w211:string)  [unwired: 8 in]
        n65 = call "Get CD source file path.vi"("CD Wizard - Internal Data"=w201) -> ("CD Source file path"=w206:path)  [unwired: 2 in]
        n66 = Merge Errors(w209, w207) -> (w208:errorcluster)
        n67 = Format Into String(format string=w211, error in=w208, w216) -> (resulting string=w214:string, error out=w202:errorcluster)  [unwired: 1 in]
        n68 = Build Path(base path=w206, name or relative path=w210) -> (appended path=w215:path)
        n69 = Build Path(base path=w215, name or relative path=w214) -> (appended path=w203:path)
        n70 = invoke class="App" method="Library.Create"(error in=w202) -> (error out=w205:errorcluster, "Create Library"=w204:refnum<vi>)  [unwired: 3 in, 2 out]
        n71 = invoke class="Library" method="Save"(reference=w204, error in=w205, "Path"=w203) -> (reference out=w199:refnum<vi>, error out=w197:errorcluster)  [unwired: 1 in, 2 out]
        n72 = Bundle By Name(cluster=w201, "References.Shared Library"=w199) -> (w200:T1)
      }
      frame "PC-Shared - Add folders and VIs to library" {
        w235 = FALSE  # Stopp?
        w248 = T13 "Folder" ("Add Item - Type")
        # "Add virtual folders and all VIs (constants.vi and CompiledSettings.ctl) to <CD> Shared.lvlib."
        n73 = Unbundle By Name(w242) -> ("References.Shared Library"=w244:refnum<vi>)
        n74 = call-poly "Constants Main.vi"("error in (no error)"=w241, "Action"=CD_Shared_lvlib."Shared.Constants.VIName") -> ("error out"=w227:errorcluster, "Output"=w263:string)  [unwired: 8 in]
        n75 = call-poly "Constants Main.vi"("error in (no error)"=w241, "Action"=CD_Shared_lvlib."Shared.FolderName") -> ("error out"=w259:errorcluster, "Output"=w237:string)  [unwired: 8 in]
        n76 = call-poly "Constants Main.vi"("error in (no error)"=w227, "Action"=CD_Shared_lvlib."Shared.CompiledSettings.Name") -> ("error out"=w226:errorcluster, "Output"=w225:string)  [unwired: 8 in]
        n77 = call-poly "Constants Main.vi"("error in (no error)"=w227, "Action"=CD_Shared_lvlib."LibraryFolderName") -> ("error out"=w238:errorcluster, "Output"=w236:string)  [unwired: 8 in]
        n78 = call-poly "Constants Main.vi"("error in (no error)"=w259, "Action"=CD_Shared_lvlib."Shared.Types.FolderName") -> ("error out"=w261:errorcluster, "Output"=w258:string)  [unwired: 8 in]
        n79 = call "Get CD source file path.vi"("CD Wizard - Internal Data"=w242) -> ("CD Source file path"=w264:path)  [unwired: 2 in]
        n80 = Merge Errors(w226, w238, w261) -> (w262:errorcluster)
        n81 = Build Path(base path=w264, name or relative path=w236) -> (appended path=w232:path)
        n82 = invoke class="Library" method="AddItem"(reference=w244, error in=w262, "Name"=w237, "Path"=path "", "Type"=w248) -> (reference out=w250:refnum<vi>, error out=w245:errorcluster, "AddItem"=w247:refnum<vi>)  [unwired: 1 in, 3 out]
        n83 = Build Path(base path=w232, name or relative path=w263) -> (appended path=w251:path)
        n84 = invoke class="ProjectItem" method="AddItem"(reference=w247, error in=w245, "Name"=w258, "Path"=path "", "Type"=w248) -> (reference out=w249:refnum<vi>, error out=w233:errorcluster, "AddItem"=w234:refnum<vi>)  [unwired: 1 in, 3 out]
        n85 = Build Path(base path=w232, name or relative path=w225) -> (appended path=w231:path)
        n86 = invoke class="ProjectItem" method="AddFile"(reference=w249, error in=w233, "Path"=w251) -> (reference out=w254:refnum<vi>, error out=w253:errorcluster)  [unwired: 1 in, 2 out]
        n87 = invoke class="ProjectItem" method="AddFile"(reference=w234, error in=w233, "Path"=w231) -> (reference out=w223:refnum<vi>, error out=w222:errorcluster)  [unwired: 1 in, 2 out]
        n88 = Close Reference(reference=w254, error in (no error)=w253) -> (error out=w255:errorcluster)
        n89 = Close Reference(reference=w223, error in (no error)=w222) -> (error out=w224:errorcluster)
        n90 = call "Save VI by path.vi"("error in (no error)"=w255, "VI path"=w251) -> ("error out"=w252:errorcluster)  [unwired: 9 in]
        n91 = call "Save VI by path.vi"("error in (no error)"=w224, "VI path"=w231) -> ("error out"=w229:errorcluster)  [unwired: 9 in]
        n92 = Merge Errors(w252, w229) -> (w230:errorcluster)
        n93 = invoke class="Library" method="Save"(reference=w250, error in=w230) -> (error out=w240:errorcluster)  [unwired: 2 in, 3 out]
      }
      frame "PC-System Explorer - Create folder and copy templates" {
        w272 = FALSE  # Stopp?
        # "Create a new folder on the file system, copy the templates and disconnect the templates from the source library."
        n94 = call-poly "Constants Main.vi"("error in (no error)"=w278, "Action"=CD_System_Explorer_lvlib."LibraryFolderName") -> ("error out"=w277:errorcluster, "Output"=w279:string)  [unwired: 8 in]
        n95 = Unbundle By Name(w271) -> ("Common Information.CD Name"=w270:string)
        n96 = call "Get CD source file path.vi"("CD Wizard - Internal Data"=w271) -> ("CD Source file path"=w273:path)  [unwired: 2 in]
        n97 = Build Path(base path=w273, name or relative path=w279) -> (appended path=w281:path)
        n98 = Create Folder(path (use dialog)=w281, error in=w277) -> (created path=w275:path, error out=w276:errorcluster)  [unwired: 1 in, 1 out]
        n99 = call "System Explorer - Copy Templates for System Explorer.vi"("CD Name"=w270, "error in (no error)"=w276, "System Explorer folder"=w275) -> ("error out"=w274:errorcluster)  [unwired: 8 in]
      }
      frame "PC-System Explorer - Create extra pages" {
        w288 = FALSE  # Stopp?
        # "Create a VI for each extra page on the file system."
        n100 = disable-structure shown="Enabled" {
          disable-tunnel: [w310 w312] -> w297
          disable-tunnel: [w307 w311] -> w290
          disable-tunnel: w289 -> [w306 w316]
          frame Disabled {
            n101 = call-poly "Constants Main.vi"("error in (no error)"=w306, "Action"=CD_System_Explorer_lvlib."System Explorer.Dynamically Called.Extra Pages.TemplatePathAndName") -> ("error out"=w307:errorcluster, "Output"=w308:string)  [unwired: 8 in]
            n102 = String To Path(string=w308) -> (path=w310:path)
          }
          frame Enabled {
            n103 = call-poly "Constants Main.vi"("error in (no error)"=w316, "Action"=Common."PathToTemplates") -> ("error out"=w311:errorcluster, "Output"=w315:string)  [unwired: 8 in]
            n104 = String To Path(string=w315) -> (path=w314:path)
            n105 = Build Path(base path=w314, name or relative path="Extra Page.vi") -> (appended path=w312:path)
          }
        }
        n106 = Unbundle By Name(w298) -> ("Common Information.CD Name"=w287:string, "Extra Pages"=w300:T3[])
        n107 = call "Get CD source file path.vi"("CD Wizard - Internal Data"=w298) -> ("CD Source file path"=w294:path)  [unwired: 2 in]
        n108 = call-poly "Constants Main.vi"("error in (no error)"=w289, "Action"=CD_System_Explorer_lvlib."LibraryFolderName") -> ("error out"=w292:errorcluster, "Output"=w296:string)  [unwired: 8 in]
        n109 = Merge Errors(w292, w290) -> (w291:errorcluster)
        n110 = Build Path(base path=w294, name or relative path=w296) -> (appended path=w293:path)
        n111 = for {
          tunnel: w300 -> [w335] mode=indexing
          shift-right: [w323] -> w299
          shift-left: w291 -> [w332]
          tunnel: w293 -> [w330]
          tunnel: w297 -> [w331]
          tunnel: w287 -> [w327]
          # "Iterate over all extra pages"
          n112 = Unbundle By Name(w335) -> ("Page Name"=w320:string)
          n113 = Concatenate Strings(w320, ".vi") -> (w333:string)
          n114 = Build Path(base path=w330, name or relative path=w333) -> (appended path=w325:path)
          n115 = Concatenate Strings(w327, ".chm" ("string")) -> (w322:string)
          n116 = call "Copy VI and disconnect it from library.vi"("error in (no error)"=w332, "VI Target Path"=w325, "VI Source Path"=w331) -> ("error out"=w329:errorcluster)  [unwired: 8 in]
          n117 = Concatenate Strings(w320, ".html" ("string")) -> (w319:string)
          n118 = call "Set BD string constant value.vi"("error in (no error)"=w329, "Name of string constant"="CD_CHM_FileName", "New String Value"=w322, "Path to VI"=w325) -> ("error out"=w326:errorcluster)  [unwired: 7 in]
          n119 = call "Set BD string constant value.vi"("error in (no error)"=w326, "Name of string constant"="CD_CHM_Section", "New String Value"=w319, "Path to VI"=w325) -> ("error out"=w323:errorcluster)  [unwired: 7 in]
        }
      }
      frame "PC-System Explorer - Create library" {
        w336 = FALSE  # Stopp?
        # "Create the library for System Explorer components."
        n120 = Unbundle By Name(w343) -> ("Common Information.CD Name"=w356:string)
        n121 = call-poly "Constants Main.vi"("error in (no error)"=w345, "Action"=CD_System_Explorer_lvlib."LibraryFolderName") -> ("error out"=w351:errorcluster, "Output"=w352:string)  [unwired: 8 in]
        n122 = call-poly "Constants Main.vi"("error in (no error)"=w345, "Action"=CD_System_Explorer_lvlib."LibraryFileName") -> ("error out"=w349:errorcluster, "Output"=w353:string)  [unwired: 8 in]
        n123 = call "Get CD source file path.vi"("CD Wizard - Internal Data"=w343) -> ("CD Source file path"=w344:path)  [unwired: 2 in]
        n124 = Merge Errors(w351, w349) -> (w350:errorcluster)
        n125 = Format Into String(format string=w353, error in=w350, w356) -> (resulting string=w354:string, error out=w338:errorcluster)  [unwired: 1 in]
        n126 = Build Path(base path=w344, name or relative path=w352) -> (appended path=w355:path)
        n127 = Build Path(base path=w355, name or relative path=w354) -> (appended path=w339:path)
        n128 = invoke class="App" method="Library.Create"(error in=w338) -> (error out=w342:errorcluster, "Create Library"=w341:refnum<vi>)  [unwired: 3 in, 2 out]
        n129 = invoke class="Library" method="Save"(reference=w341, error in=w342, "Path"=w339) -> (reference out=w340:refnum<vi>, error out=w337:errorcluster)  [unwired: 1 in, 2 out]
        n130 = Bundle By Name(cluster=w343, "References.System Explorer Library"=w340) -> (w346:T1)
      }
      frame "PC-System Explorer - Add folders and VIs to library" {
        w362 = FALSE  # Stopp?
        # "Add virtual folders and all VIs to <CD> System Explorer.lvlib"
        n131 = call "System Explorer - Add content to System Explorer library.vi"("error in (no error)"=w365, "CD Wizard - Internal Data IN"=w363) -> ("error out"=w364:errorcluster)  [unwired: 9 in]
      }
      frame "PC-Engine - Create folder and copy the RT Template" {
        w382 = FALSE  # Stopp?
        # "Create a new Engine folder on the file system and copy the RT Driver VI for the chosen custom device."
        n132 = call-poly "Constants Main.vi"("error in (no error)"=w383, "Action"=CD_Engine_lvlib."LibraryFolderName") -> ("error out"=w388:errorcluster, "Output"=w390:string)  [unwired: 8 in]
        n133 = call "Get CD source file path.vi"("CD Wizard - Internal Data"=w387) -> ("CD Source file path"=w371:path)  [unwired: 2 in]
        n134 = call-poly "Constants Main.vi"("error in (no error)"=w388, "Action"=CD_Engine_lvlib."Engine.RT Driver VI.FileName") -> ("error out"=w375:errorcluster, "Output"=w379:string)  [unwired: 8 in]
        n135 = Build Path(base path=w371, name or relative path=w390) -> (appended path=w392:path)
        n136 = Create Folder(path (use dialog)=w392, error in=w375) -> (created path=w372:path, error out=w386:errorcluster)  [unwired: 1 in, 1 out]
        n137 = call-poly "Constants Main.vi"("error in (no error)"=w386, "Action"=Common."ProjectTemplatePathAndName") -> ("error out"=w384:errorcluster, "Output"=w380:string)  [unwired: 8 in]
        n138 = String To Path(string=w380) -> (path=w381:path)
        n139 = Build Path(base path=w372, name or relative path=w379) -> (appended path=w373:path)
        n140 = Strip Path(path=w381) -> (stripped path=w377:path)  [unwired: 1 out]
        n141 = Build Path(base path=w377, name or relative path=w379) -> (appended path=w385:path)
        n142 = call "Copy VI and disconnect it from library.vi"("error in (no error)"=w384, "VI Target Path"=w373, "VI Source Path"=w385) -> ("error out"=w376:errorcluster)  [unwired: 8 in]
        n143 = call "Engine - Copy & Script Templates.vi"("error in (no error)"=w376, "RT Driver VI Path"=w373, "RT Driver Folder Path"=w372, "CD Source Folder Path"=w371) -> ("error out"=w374:errorcluster)  [unwired: 7 in]
      }
      frame "PC-Engine - Create library" {
        w398 = FALSE  # Stopp?
        # "Create the library for the Engine components."
        n144 = Unbundle By Name(w407) -> ("Common Information.CD Name"=w418:string)
        n145 = call-poly "Constants Main.vi"("error in (no error)"=w405, "Action"=CD_Engine_lvlib."LibraryFolderName") -> ("error out"=w413:errorcluster, "Output"=w414:string)  [unwired: 8 in]
        n146 = call-poly "Constants Main.vi"("error in (no error)"=w405, "Action"=CD_Engine_lvlib."LibraryFileName") -> ("error out"=w411:errorcluster, "Output"=w415:string)  [unwired: 8 in]
        n147 = Merge Errors(w413, w411) -> (w412:errorcluster)
        n148 = Format Into String(format string=w415, error in=w412, w418) -> (resulting string=w416:string, error out=w402:errorcluster)  [unwired: 1 in]
        n149 = call "Get CD source file path.vi"("CD Wizard - Internal Data"=w407) -> ("CD Source file path"=w410:path)  [unwired: 2 in]
        n150 = Build Path(base path=w410, name or relative path=w414) -> (appended path=w417:path)
        n151 = Build Path(base path=w417, name or relative path=w416) -> (appended path=w399:path)
        n152 = invoke class="App" method="Library.Create"(error in=w402) -> (error out=w404:errorcluster, "Create Library"=w403:refnum<vi>)  [unwired: 3 in, 2 out]
        n153 = invoke class="Library" method="Save"(reference=w403, error in=w404, "Path"=w399) -> (reference out=w400:refnum<vi>, error out=w401:errorcluster)  [unwired: 1 in, 2 out]
        n154 = Bundle By Name(cluster=w407, "References.Engine Library"=w400) -> (w406:T1)
      }
      frame "PC-Engine - Add virtual folders and VIs to library" {
        w424 = FALSE  # Stopp?
        # "Add all virtual folders and template VIs to the Engine library"
        n155 = call "Engine - Add content to Engine library.vi"("error in (no error)"=w427, "CD Wizard - Internal Data IN"=w425) -> ("error out"=w426:errorcluster)  [unwired: 9 in]
      }
      frame "PC-XML - Create and change file" {
        w433 = FALSE  # Stopp?
        # "Create the XML file and add it to the project tree"
        n156 = call "XML - Create XML file.vi"("error in (no error)"=w436, "CD Wizard - Internal Data"=w434) -> ("error out"=w435:errorcluster)  [unwired: 8 in, 1 out]
      }
      frame "PC-Help - Copy HTML Files" {
        w455 = "Main"
        w470 = "OPTIONS" ("section")
        # "Note: We only copy the files here, the get added to the project in the \"Write New Project File\" case since\nthe project doesn't exist (to add the folder to) until that case."
        # "Copy all of the HTML template files to the new help directory, and configure Build CHM file."
        n157 = Unbundle By Name(w452) -> ("Common Information.CD Name"=w450:string, "Extra Pages"=w449:T3[])
        n158 = call "Get CD source file path.vi"("CD Wizard - Internal Data"=w452) -> ("CD Source file path"=w451:path)  [unwired: 2 in]
        n159 = Build Path(base path=w451, name or relative path="Help") -> (appended path=w454:path)
        n160 = call <vilib>:"Check if File or Folder Exists.vi"("error in (no error)"=w457, "path"=w454) -> ("error out"=w463:errorcluster, "file or folder exists?"=w477:bool, "dup path"=w478:path)  [unwired: 7 in]
        n161 = for {
          tunnel: w449 -> [w486] mode=indexing
          tunnel: [w485] -> w448 mode=indexing
          n162 = Unbundle By Name(w486) -> ("Page Name"=w485:string)
        }
        n163 = case shown="False" w477 {
          tunnel: w478 -> [w488 w492]
          tunnel: [w488 w491] -> w445
          tunnel: [w487 w490] -> w464
          tunnel: w463 -> [w487 w489]
          frame False {
          }
          frame True {
            n164 = Delete(path (use dialog)=w492, entire hierarchy (F)=TRUE, error in=w489) -> (deleted path=w491:path, error out=w490:errorcluster)  [unwired: 2 in, 1 out]
          }
        }
        n165 = Build Array (concatenate)(w455, w448) -> (w444:string[])
        n166 = Concatenate Strings("HTML Help Source\\" ("string"), w455, ".htm" ("string")) -> (w459:string)
        n167 = Create Folder(path (use dialog)=w445, error in=w464) -> (created path=w447:path, error out=w446:errorcluster)  [unwired: 1 in, 1 out]
        n168 = call "Call HTML Help Generation Functions Async.vi"("error in (no error)"=w446, "Extra Page Names"=w444, "Destination Base Path"=w447) -> ("error out"=w443:errorcluster, "Destination Base Path Out (dup)"=w442:path)  [unwired: 7 in]
        n169 = Build Path(base path=w447, name or relative path="Build CHM.cfg") -> (appended path=w461:path)
        n170 = call <vilib>:"Open Config Data.vi"("error in (no error)"=w443, "configuration file path"=w461) -> ("error out"=w476:errorcluster, "refnum"=w475:T14)  [unwired: 7 in, 1 out]
        n171 = call-poly <vilib>:"Write Key.vi"("section"=w470, "error in (no error)"=w476, "value"=w450, "key"="Title", "refnum"=w475) -> ("error out"=w473:errorcluster, "refnum out"=w472:T14)  [unwired: 4 in, 1 out]
        n172 = call-poly <vilib>:"Write Key.vi"("section"=w470, "error in (no error)"=w473, "value"=w459, "key"="Default Topic", "refnum"=w472) -> ("error out"=w469:errorcluster, "refnum out"=w467:T14)  [unwired: 4 in, 1 out]
        n173 = call-poly <vilib>:"Write Key.vi"("section"=w470, "error in (no error)"=w469, "value"=w442, "key"="Base Path", "refnum"=w467) -> ("error out"=w468:errorcluster, "refnum out"=w466:T14)  [unwired: 4 in, 1 out]
        n174 = call <vilib>:"Close Config Data.vi"("error in (no error)"=w468, "refnum"=w466) -> ("error out"=w456:errorcluster)  [unwired: 8 in, 1 out]
      }
      frame "Project - Read project file content" {
        w494 = FALSE  # Stopp?
        w507 = -1  # Read all lines
        w506 = T12."open"  # operation
        w505 = enum16{"read/write", "read-only", "write-only"}."read-only"  # access
        # "Open the project file and read the complete content."
        n175 = call-poly "Constants Main.vi"("error in (no error)"=w497, "Action"=Common."ProjectTemplatePathAndName") -> ("Output"=w498:string)  [unwired: 8 in, 1 out]
        n176 = String To Path(string=w498) -> (path=w499:path)
        n177 = Open/Create/Replace File(file path (use dialog)=w499, error in=w497, operation (0:open)=w506, access (0:read/write)=w505) -> (refnum out=w503:refnum<file>, error out=w504:errorcluster)  [unwired: 3 out]
        n178 = Read from Text File(file (use dialog)=w503, count=w507, error in=w504) -> (refnum out=w496:refnum<file>, text=w501:string[], error out=w502:errorcluster)  [unwired: 2 out]
        n179 = Close File(refnum=w496) -> ()  [unwired: 1 in, 2 out]
      }
      frame "Project - Edit Utility section" {
        w518 = FALSE  # Stopp?
        # "Also added CHM pre build action entries"
        # "Edit the entries for the utility folder."
        n180 = call-poly "Constants Main.vi"("error in (no error)"=w516, "Action"=Utility_folder."Utility.Copy .llb to NI VeriStand dir.FileName") -> ("error out"=w525:errorcluster, "Output"=w521:string)  [unwired: 8 in]
        n181 = call-poly "Constants Main.vi"("error in (no error)"=w516, "Action"=Utility_folder."Utility.FolderName") -> ("error out"=w524:errorcluster, "Output"=w520:string)  [unwired: 8 in]
        n182 = call-poly "Constants Main.vi"("error in (no error)"=w516, "Action"=Utility_folder."Utility.LLB Pre Build.FilePathAndName") -> ("error out"=w515:errorcluster, "Output"=w514:string)  [unwired: 8 in]
        n183 = Merge Errors(w524, w525, w515) -> (w519:errorcluster)
        n184 = String To Path(string=w514) -> (path=w513:path)
        n185 = Strip Path(path=w513) -> (name=w512:string)  [unwired: 1 out]
        n186 = for {
          tunnel: w528 -> [w544] mode=indexing
          shift-right: [w540] -> w526
          shift-left: w519 -> [w542]
          tunnel: [w538] -> w527 mode=indexing
          tunnel: w521 -> [w543]
          tunnel: w520 -> [w541]
          tunnel: w512 -> [w534]
          w536 = TRUE  # ignore case? (F)
          w537 = TRUE  # replace all? (F)
          w547 = "%CopyLLBtoNIVSFileName%"  # search
          w549 = "%UtilityFolderName%"  # search
          # "CHM Build VI as pre-build action"
          # "Copy .LLB to NI VeriStand dir.vi"
          # "Utility"
          # "Iterate over each line and change the placeholders for the Utility entries."
          n187 = Search and Replace String(replace all?=w537, case sensitive?=w536, input string=w544, search string=w549, replace string=w541, error in=w542) -> (result string=w548:string, error out=w546:errorcluster)  [unwired: 2 in, 2 out]
          n188 = Search and Replace String(replace all?=w537, case sensitive?=w536, input string=w548, search string=w547, replace string=w543, error in=w546) -> (result string=w539:string, error out=w545:errorcluster)  [unwired: 2 in, 2 out]
          n189 = Search and Replace String(replace all?=w537, case sensitive?=w536, input string=w539, search string="%CHMPreBuild%" ("result string"), replace string=w534, error in=w545) -> (result string=w538:string, error out=w540:errorcluster)  [unwired: 2 in, 2 out]
        }
      }
      frame "Project - Edit XML section" {
        w550 = FALSE  # Stopp?
        # "Edit the Name and Path for the XML file."
        n190 = Unbundle By Name(w556) -> ("Common Information.CD Name"=w552:string, "Common Information.CD Execution Mode"=w551:T2)
        n191 = call "XML - Get XML file name.vi"("error in (no error)"=w555, "CD Execution Mode (Asynchronous)"=w551, "CD Name"=w552) -> ("error out"=w554:errorcluster, "XML file name"=w553:string)  [unwired: 7 in]
        n192 = for {
          tunnel: w558 -> [w570] mode=indexing
          shift-right: [w569] -> w559
          shift-left: w554 -> [w565]
          tunnel: [w568] -> w557 mode=indexing
          tunnel: w553 -> [w564]
          w566 = TRUE  # ignore case? (F)
          w567 = TRUE  # replace all? (F)
          w571 = "%XMLCustomDeviceFileName%"  # search
          # "Iterate over each line and change the placeholder for the XML file name."
          n193 = Search and Replace String(replace all?=w567, case sensitive?=w566, input string=w570, search string=w571, replace string=w564, error in=w565) -> (result string=w568:string, error out=w569:errorcluster)  [unwired: 2 in, 2 out]
        }
      }
      frame "Project - Edit Engine Library section" {
        w572 = FALSE  # Stopp?
        # "Edit the entries for the Engine Library (Library name and folder name)"
        n194 = call "Change Engine Library Placeholders in project.vi"("error in (no error)"=w576, "CD Wizard - Internal Data"=w574, "Project file content IN"=w573) -> ("error out"=w575:errorcluster, "Project file content OUT"=w577:string[])  [unwired: 7 in]
      }
      frame "Project - Edit Shared Library section" {
        w582 = FALSE  # Stopp?
        # "Edit the entries for the Shared Library (Library name and folder name)"
        n195 = Unbundle By Name(w583) -> ("Common Information.CD Name"=w593:string)
        n196 = call-poly "Constants Main.vi"("error in (no error)"=w587, "Action"=CD_Shared_lvlib."LibraryFileName") -> ("error out"=w592:errorcluster, "Output"=w591:string)  [unwired: 8 in]
        n197 = call-poly "Constants Main.vi"("error in (no error)"=w587, "Action"=CD_Shared_lvlib."LibraryFolderName") -> ("error out"=w597:errorcluster, "Output"=w585:string)  [unwired: 8 in]
        n198 = call-poly "Constants Main.vi"("error in (no error)"=w587, "Action"=CD_Shared_lvlib."Shared.FolderName") -> ("error out"=w598:errorcluster, "Output"=w584:string)  [unwired: 8 in]
        n199 = Format Into String(format string=w591, error in=w592, w593) -> (resulting string=w586:string, error out=w596:errorcluster)  [unwired: 1 in]
        n200 = Merge Errors(w596, w597, w598) -> (w589:errorcluster)
        n201 = for {
          tunnel: w588 -> [w619] mode=indexing
          shift-right: [w612] -> w599
          shift-left: w589 -> [w618]
          tunnel: [w613] -> w600 mode=indexing
          tunnel: w586 -> [w607]
          tunnel: w585 -> [w606]
          tunnel: w584 -> [w605]
          w610 = "%SharedLibrarySubfolderName%"  # search
          w616 = "%SharedLibraryFolderName%"  # search
          w608 = TRUE  # ignore case? (F)
          w609 = TRUE  # replace all? (F)
          w620 = "%SharedLibraryFileName%"  # search
          # "Shared"
          # "Shared"
          # "<CD> Shared.lvlib"
          # "Iterate over each line and change the placeholder for the Shared Library file and folder name."
          n202 = Search and Replace String(replace all?=w609, case sensitive?=w608, input string=w619, search string=w620, replace string=w607, error in=w618) -> (result string=w617:string, error out=w615:errorcluster)  [unwired: 2 in, 2 out]
          n203 = Search and Replace String(replace all?=w609, case sensitive?=w608, input string=w617, search string=w616, replace string=w606, error in=w615) -> (result string=w614:string, error out=w611:errorcluster)  [unwired: 2 in, 2 out]
          n204 = Search and Replace String(replace all?=w609, case sensitive?=w608, input string=w614, search string=w610, replace string=w605, error in=w611) -> (result string=w613:string, error out=w612:errorcluster)  [unwired: 2 in, 2 out]
        }
      }
      frame "Project - Edit System Explorer Library section" {
        w621 = FALSE  # Stopp?
        # "Edit the entries for the System Explorer Library (Library name and folder name)"
        n205 = Unbundle By Name(w623) -> ("Common Information.CD Name"=w630:string)
        n206 = call-poly "Constants Main.vi"("error in (no error)"=w622, "Action"=CD_System_Explorer_lvlib."LibraryFolderName") -> ("error out"=w634:errorcluster, "Output"=w638:string)  [unwired: 8 in]
        n207 = call-poly "Constants Main.vi"("error in (no error)"=w622, "Action"=CD_System_Explorer_lvlib."LibraryFileName") -> ("error out"=w629:errorcluster, "Output"=w628:string)  [unwired: 8 in]
        n208 = call-poly "Constants Main.vi"("error in (no error)"=w622, "Action"=CD_System_Explorer_lvlib."System Explorer.FolderName") -> ("error out"=w633:errorcluster, "Output"=w639:string)  [unwired: 8 in]
        n209 = Format Into String(format string=w628, error in=w629, w630) -> (resulting string=w637:string, error out=w635:errorcluster)  [unwired: 1 in]
        n210 = Merge Errors(w635, w634, w633) -> (w636:errorcluster)
        n211 = for {
          tunnel: w624 -> [w658] mode=indexing
          shift-right: [w650] -> w626
          shift-left: w636 -> [w657]
          tunnel: [w651] -> w625 mode=indexing
          tunnel: w637 -> [w646]
          tunnel: w638 -> [w645]
          tunnel: w639 -> [w644]
          w647 = "%SystemExplorerSubfolderName%"  # search
          w655 = "%SystemExplorerLibraryFolderName%"  # search
          w649 = TRUE  # ignore case? (F)
          w648 = TRUE  # replace all? (F)
          w659 = "%SystemExplorerLibraryFileName%"  # search
          # "System Explorer"
          # "System Explorer"
          # "<CD> System Explorer.lvlib"
          # "Iterate over each line and change the placeholder for the System Explorer Library file and folder name."
          n212 = Search and Replace String(replace all?=w648, case sensitive?=w649, input string=w658, search string=w659, replace string=w646, error in=w657) -> (result string=w656:string, error out=w654:errorcluster)  [unwired: 2 in, 2 out]
          n213 = Search and Replace String(replace all?=w648, case sensitive?=w649, input string=w656, search string=w655, replace string=w645, error in=w654) -> (result string=w652:string, error out=w653:errorcluster)  [unwired: 2 in, 2 out]
          n214 = Search and Replace String(replace all?=w648, case sensitive?=w649, input string=w652, search string=w647, replace string=w644, error in=w653) -> (result string=w651:string, error out=w650:errorcluster)  [unwired: 2 in, 2 out]
        }
      }
      frame "Project - Edit Custom Device Name" {
        w660 = FALSE  # Stopp?
        # "Edit the Custom Device name"
        n215 = Unbundle By Name(w661) -> ("Common Information.CD Name"=w662:string)
        n216 = for {
          tunnel: w663 -> [w677] mode=indexing
          shift-right: [w672] -> w665
          shift-left: w666 -> [w673]
          tunnel: [w676] -> w664 mode=indexing
          tunnel: w662 -> [w671]
          w674 = TRUE  # ignore case? (F)
          w675 = TRUE  # replace all? (F)
          w678 = "%CustomDeviceName%"  # search
          # "<CD>"
          # "Iterate over each line and change the placeholder for the Custom Device name."
          n217 = Search and Replace String(replace all?=w675, case sensitive?=w674, input string=w677, search string=w678, replace string=w671, error in=w673) -> (result string=w676:string, error out=w672:errorcluster)  [unwired: 2 in, 2 out]
        }
      }
      frame "Project - Edit System Explorer LLB Name" {
        w679 = FALSE  # Stopp?
        # "Edit the name for the System Explorer LLB."
        n218 = Unbundle By Name(w684) -> ("Common Information.CD Name"=w683:string)
        n219 = call-poly "Constants Main.vi"("error in (no error)"=w686, "Action"=Build_Spec_System_Explorer."Destinations.LLBFileName") -> ("error out"=w688:errorcluster, "Output"=w689:string)  [unwired: 8 in]
        n220 = Format Into String(format string=w689, error in=w688, w683) -> (resulting string=w682:string, error out=w685:errorcluster)  [unwired: 1 in]
        n221 = for {
          tunnel: w682 -> [w700]
          tunnel: w681 -> [w698] mode=indexing
          tunnel: [w697] -> w680 mode=indexing
          shift-right: [w696] -> w690
          shift-left: w685 -> [w699]
          w695 = "%SystemExplorerLLBFileName%"  # search
          w701 = TRUE  # ignore case? (F)
          w702 = TRUE  # replace all? (F)
          # "<CD> Configuration.llb"
          # "Iterate over each line and change the placeholder for the System Explorer LLB."
          n222 = Search and Replace String(replace all?=w702, case sensitive?=w701, input string=w698, search string=w695, replace string=w700, error in=w699) -> (result string=w697:string, error out=w696:errorcluster)  [unwired: 1 in, 3 out]
        }
      }
      frame "Project - Edit Engine LLB OS dependent file name" {
        w720 = FALSE  # Stopp?
        n223 = Unbundle By Name(w733) -> ("Common Information.CD Name"=w713:string)
        n224 = call-poly "Constants Main.vi"("error in (no error)"=w712, "Action"=Build_Spec_Engine."Destinations.LLBWindowsFileName") -> ("error out"=w735:errorcluster, "Output"=w736:string)  [unwired: 8 in]
        n225 = call-poly "Constants Main.vi"("error in (no error)"=w712, "Action"=Build_Spec_Engine."Destinations.LLBVxWorksFileName") -> ("error out"=w731:errorcluster, "Output"=w730:string)  [unwired: 8 in]
        n226 = call-poly "Constants Main.vi"("error in (no error)"=w712, "Action"=Build_Spec_Engine."Destinations.LLBLinux64FileName") -> ("error out"=w715:errorcluster, "Output"=w716:string)  [unwired: 8 in]
        n227 = call-poly "Constants Main.vi"("error in (no error)"=w712, "Action"=Build_Spec_Engine."Destinations.LLBLinuxARMFileName") -> ("error out"=w718:errorcluster, "Output"=w717:string)  [unwired: 8 in]
        n228 = call-poly "Constants Main.vi"("error in (no error)"=w712, "Action"=Build_Spec_Engine."Destinations.LLBPharlapFileName") -> ("error out"=w728:errorcluster, "Output"=w729:string)  [unwired: 8 in]
        n229 = Format Into String(format string=w716, error in=w715, w713) -> (resulting string=w705:string, error out=w711:errorcluster)  [unwired: 1 in]
        n230 = Format Into String(format string=w717, error in=w718, w713) -> (resulting string=w706:string, error out=w710:errorcluster)  [unwired: 1 in]
        n231 = Format Into String(format string=w736, error in=w735, w713) -> (resulting string=w709:string, error out=w724:errorcluster)  [unwired: 1 in]
        n232 = Format Into String(format string=w730, error in=w731, w713) -> (resulting string=w708:string, error out=w725:errorcluster)  [unwired: 1 in]
        n233 = Format Into String(format string=w729, error in=w728, w713) -> (resulting string=w707:string, error out=w726:errorcluster)  [unwired: 1 in]
        n234 = Build Array(w709, w708, w707, w706, w705) -> (w704:string[])
        n235 = Merge Errors(w724, w725, w726, w710, w711) -> (w723:errorcluster)
        n236 = for {
          shift-right: [w745] -> w721
          shift-left: w723 -> [w746]
          tunnel: w722 -> [w742] mode=indexing
          tunnel: w704 -> [w743]
          tunnel: [w741] -> w703 mode=indexing
          n237 = for {
            shift-right: [w754] -> w745
            shift-left: w746 -> [w753]
            shift-right: [w750] -> w741
            shift-left: w742 -> [w749]
            tunnel: string[] ["%EngineLLBWindowsFileName%", "%EngineLLBVxWorksFileName%", "%EngineLLBPharlapFileName%", "%EngineLLBLinuxARMFileName%", "%EngineLLBLinux64FileName%"] -> [w748] mode=indexing
            tunnel: w743 -> [w747] mode=indexing
            w751 = TRUE  # ignore case? (F)
            w752 = TRUE  # replace all? (F)
            n238 = Search and Replace String(replace all?=w752, case sensitive?=w751, input string=w749, search string=w748, replace string=w747, error in=w753) -> (result string=w750:string, error out=w754:errorcluster)  [unwired: 1 in, 3 out]
          }
        }
      }
      frame "Project - Write new project file" {
        w770 = FALSE  # Stopp?
        # "Create new file and write the project file content into it."
        n239 = Unbundle By Name(w783) -> ("Common Information.CD Name"=w787:string)
        n240 = call "Get CD source file path.vi"("CD Wizard - Internal Data"=w783) -> ("CD Source file path"=w757:path)  [unwired: 2 in]
        n241 = call-poly "Constants Main.vi"("error in (no error)"=w782, "Action"=Common."ProjectName") -> ("error out"=w784:errorcluster, "Output"=w771:string)  [unwired: 8 in]
        n242 = Format Into String(format string=w771, error in=w784, w787) -> (resulting string=w786:string, error out=w778:errorcluster)  [unwired: 1 in]
        n243 = Build Path(base path=w757, name or relative path=w786) -> (appended path=w779:path)
        n244 = Build Path(base path=w757, name or relative path="Help") -> (appended path=w755:path)
        n245 = Open/Create/Replace File(file path (use dialog)=w779, error in=w778, operation (0:open)=T12."replace or create") -> (refnum out=w781:refnum<file>, error out=w780:errorcluster)  [unwired: 3 in, 1 out]
        n246 = Write to Text File(file (use dialog)=w781, text=w775, error in=w780) -> (refnum out=w777:refnum<file>, error out=w776:errorcluster)  [unwired: 2 out]
        n247 = Close File(refnum=w777, error in=w776) -> (path=w773:path, error out=w769:errorcluster)
        n248 = invoke class="App" method="Project.Open"(error in=w769, "Path"=w773) -> (error out=w764:errorcluster, "Project:Open"=w763:refnum<vi>)  [unwired: 2 in, 2 out]
        n249 = property class="Project"(reference=w763, error in=w764) -> (reference out=w762:refnum<vi>, error out=w759:errorcluster, "My Computer"=w761:refnum<vi>)
        n250 = invoke class="TargetItem" method="AddItem"(reference=w761, error in=w759, "Name"="Placeholder", "Path"=path "", "Type"="Folder") -> (error out=w767:errorcluster, "AddItem"=w766:refnum<vi>)  [unwired: 1 in, 4 out]
        n251 = invoke class="ProjectItem" method="Convert to Auto-populating Folder"(reference=w766, error in=w767, "Path"=w755) -> (error out=w760:errorcluster)  [unwired: 1 in, 3 out]
        n252 = invoke class="Project" method="Open Window"(reference=w762, error in=w760) -> (error out=w772:errorcluster)  [unwired: 1 in, 2 out]
      }
      frame "Shutdown" {
        w792 = TRUE  # Stopp?
        # "Stop the State Machine"
      }
    }
    n253 = Or(x=w21, y=w18) -> (x .or. y?=w22:bool)
  }
  n254 = Release Queue(queue=w11, error in (no error)=w4) -> (error out=→"error out":errorcluster)  [unwired: 1 in, 2 out]
